vi "Stufen abfragen.vi"(4 "auto Scan Points":bool, 5 "Punkte umkehren":bool, 6 "Sprachliste":string[][](array[string]), 7 "Komponentenauswahl":T9 {"Konzentration" format="%#.6f"}, 8 "error in (no error)":errorcluster caption="Fehler (Eingang, kein Fehler)", 9 "Index Cluster":T7 {"Verdünnungsgas" items=["N2", "O2"]; "Anzahl Stufen" format="%#_5g"}, 10 "Bollche Flags Cluster":T2, 11 "GD Info Cluster":T1) -> (0 "error out":errorcluster caption="Fehler (Ausgang)", 1 "Komponente out":T8, 2 "Status out":string, 3 "GD out":T4)   [LabVIEW 2020, in "Linearisierung v2.lvlib" / "Gasteiler.lvlib"]
uses:
  Gasteiler.lvlib
  KomponentenArray.ctl
  Visualisierungs Elemente/Auswahlfeld.ctl
  Visualisierungs Elemente/Zahlen-Eingabefeld.ctl
  Seiten/System Einstellungen V2/Traegergas.ctl
  Aktionen FGV Gasteiler Daten.ctl
  Aktion FGV Gasteilerliste laden.ctl
  SpanEinstellungen/Aktion FGV GD Errors sammeln.ctl
  SpanEinstellungen/GD Info Cluster.ctl
  LIN ErrorCluster.ctl
  AK-Komm Gasteiler/Aktionen AK Komm.ctl
  AK-Komm Gasteiler/Alter Gasteiler/Aktionen AK Komm_ALT.ctl
  Horiba/Aktion Befehl.ctl
  Gasteiler Fehler.ctl
  Aktion FGV Gasteiler Korrektur.ctl
  AK-Komm Gasteiler/AK Komm Gasteiler.lvlib
  Aktion Lin Daten aufarbeiten.ctl
  Linearisierung v2.lvlib
  AK-Komm Gasteiler/Alter Gasteiler/Alter Gasteiler.lvlib
  Horiba/Horiba GDC.lvlib
  SpanEinstellungen/SpanEinstellungen.lvlib
  HovaCal/HovaCal.lvlib
  Seiten/System Einstellungen V2/System Einstellungen V2.lvlib
  HovaCAL_Interface/HovaCAL_Interface.lvlib
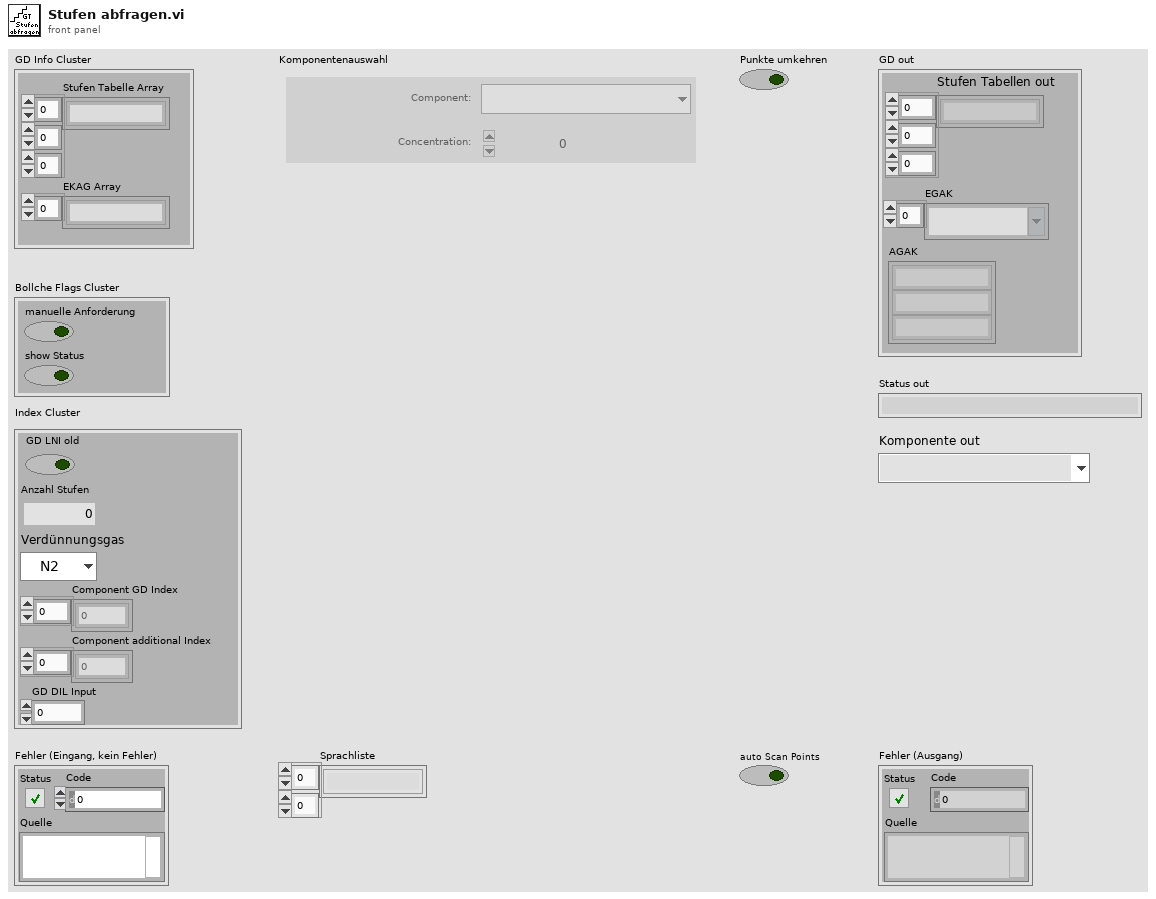
[diagram p1: front panel]
types:
  T1 = cluster{"Stufen Tabelle Array":string[][][], "EKAG Array":string[]}
  T2 = cluster{"manuelle Anforderung":bool, "show Status":bool}
  T3 = typedef "System Einstellungen V2.lvlib/Traegergas.ctl" = string
  T4 = cluster{"Stufen Tabellen out":string[][][], "EGAK":T3[], "AGAK":string[]}
  T5 = typedef "Zahlen-Eingabefeld.ctl" = sgl
  T6 = typedef "Linearisierung v2.lvlib/Gasteiler.lvlib/Prüfgas in.ctl" = u16
  T7 = cluster{"GD LNI old":bool, "Anzahl Stufen":T5, "Verdünnungsgas":T6, "Component GD Index":i32[], "Component additional Index ":i32[], "GD DIL Input":u16}
  T8 = typedef "Auswahlfeld.ctl" = u16
  T9 = typedef "Linearisierung v2.lvlib/KomponentenArray.ctl" = cluster{"Komponente:":T8, "Konzentration":dbl}[]
  T10 = typedef "Linearisierung v2.lvlib/Gasteiler.lvlib/Aktionen FGV Gasteiler Daten.ctl" = enum16{"lesen", "Gasteiler Daten", "Seriellen Param.", "MB-Endwert", "laden", "speichern", "Anforderung", "TCP", "Aufzeichnung Start"}
  T11 = typedef "Linearisierung v2.lvlib/Aktion Lin Daten aufarbeiten.ctl" = enum16{"lesen", "Protkolldaten", "speichern", "laden", "EPA auswerten", "Tabelle schreiben", "Lin auswerten", "Tab init", "Stufentabelle", "EPA aktiviert", "Nachbehandlung laden", "Tabelle löschen", "Istwerte löschen", "Zeile löschen", "Zeile einfügen", "LIN aktiviert", "LIN/EPA aktiv laden", "EGAK Tab", "LIN übernehmen", "Tab init ohne Stufen"}
  T12 = typedef "Linearisierung v2.lvlib/Lin-Polynom Daten.ctl" = cluster{"Messgerät":string, "Kalibrator (Gasteiler)":string, "Bearbeiter/in":string, "Komponente":string, "Zeitstempel":timestamp, "F_max gefordert (%)":sgl, "F_max in %":sgl, "F_max in ppm":sgl, "Vorschlag Ordnung":i32, "Polynom OK":bool, "Polynomkoeff.":dbl[], "Prüfgas Konzentration":dbl, "Pfad EPA":string, "Pfad_LIN":string, "Gasnummer:":u8, "Komponentenauswahl":T9, "Verdünnungsgas":T6, "Zeitdauer Stufe":T5, "Anzahl Stufen":T5, "F_max in % EPA":sgl, "F_max in ppm EPA":sgl, "F_max in % LIN":sgl, "F_max in ppm LIN":sgl, "Punkte umkehren":bool, "EPA Optionsfeld":T13, "Autolin Hovacal":T14, "Spanfactors":sgl[], "Kalibrierauswahl":T15, "Conditions:":T16, "Gasflaschen Nr.:":string, "Bottle Accuracy":dbl, "Konfig Gasflasche":T17, "Gasflasche":T18, "HovaCAL Flow AutoLin":T19, "MFC Output":T20, "Gas Ablaufdatum":timestamp, "Lin Modus":T21, "zusätzliche Zeitdauer Erster Punkt":sgl, "Offsets":sgl[]}
  T13 = typedef "Linearisierung v2.lvlib/EPA Optionsfeld.ctl" = enum32{"Istwert", "Rohwert", "Linearisierter Wert"}
  T14 = typedef "Linearisierung v2.lvlib/Gasteiler.lvlib/HovaCal.lvlib/AutoLin Hovacal.ctl" = enum32{"Keine Auswahl", "Optionsauswahl 1", "Optionsauswahl 2"}
  T15 = typedef "Linearisierung v2.lvlib/Kalibrieroption.ctl" = u16
  T16 = typedef "Linearisierung v2.lvlib/Linearity verification 1065-307.lvlib/Condition.ctl" = u16
  T17 = typedef "System Einstellungen V2.lvlib/Konfig Gasflasche.ctl" = bool
  T18 = typedef "System Einstellungen V2.lvlib/Gasflasche Auswahl.ctl" = u16
  T19 = typedef "Linearisierung v2.lvlib/Gasteiler.lvlib/HovaCAL_Interface.lvlib/Controls.lvlib/Flow Einstellung.ctl" = cluster{"HovaCAL Flow Input Cluster":dbl}
  T20 = typedef "Linearisierung v2.lvlib/Gasteiler.lvlib/HovaCAL_Interface.lvlib/Controls.lvlib/Pump state.ctl" = cluster{"Run":bool}
  T21 = typedef "Linearisierung v2.lvlib/Lin Modus.ctl" = u16
  T22 = typedef "Linearisierung v2.lvlib/Gasteiler.lvlib/Aktion FGV Gasteilerliste laden.ctl" = enum16{"lesen", "laden", "speichern", "Liste erstellen", "Formel ändern", "Gas vereinzeln"}
  T23 = typedef "Linearisierung v2.lvlib/Gasteiler.lvlib/Gasteiler Daten.ctl" = cluster{"Gasteiler":T24, "Gasteiler Stufen":T25, "Gasteiler Type":T26, "Konfig Gasteiler":T27, "Gasteiler Span Eingänge":u16}
  T24 = typedef "String - Eingabefeld.ctl" = string
  T25 = typedef "Linearisierung v2.lvlib/Gasteiler.lvlib/Gasteiler Stufen.ctl" = u16
  T26 = typedef "Linearisierung v2.lvlib/GasteilerType.ctl" = u16
  T27 = typedef "System Einstellungen V2.lvlib/Gasteiler Auswahl.ctl" = u16
  T28 = typedef "Linearisierung v2.lvlib/SpanEinstellungen.lvlib/GD Info Cluster.ctl" = cluster{"Wobei":string, "Status":string, "Errors":T29, "Empfangsdaten":string[], "Zeitstempel":string}
  T29 = typedef "Linearisierung v2.lvlib/LIN ErrorCluster.ctl" = cluster{"Störung Kommunikation":bool, "Pressure carrier gas":bool, "Pressure diluted gas":bool, "Outlet Pressure":bool, "SNOX before SAIR":bool, "Störung Gasteiler":bool}
  T30 = typedef "Linearisierung v2.lvlib/SpanEinstellungen.lvlib/Aktion FGV GD Errors sammeln.ctl" = enum16{"lesen", "init", "GD Infos sammeln", "Kalibrierinfos sammeln", "Test Data", "GD Infos selektiv sammeln"}
  T31 = typedef "Linearisierung v2.lvlib/Gasteiler.lvlib/AK Komm Gasteiler.lvlib/Aktionen AK Komm.ctl" = enum16{"lesen", "initialisieren", "beenden", "Status", "SMAN", "SREM", "STBY", "ASTF", "ASTZ", "SLST", "AGAT", "EGAK", "AGAK", "AKAK", "ADRU", "SKOP", "SVSA", "SVSZ", "SONO", "SAIR", "SNOX", "ANOX", "SSPL", "SRUC", "SLIN", "ALST", "ETYP", "SVIO", "LCYL", "CCYL", "DCYL", "SCYL", "GCYL", "DRGV", "DRDC"}
  T32 = typedef "Linearisierung v2.lvlib/Gasteiler.lvlib/AK Komm Gasteiler.lvlib/Alter Gasteiler.lvlib/Aktionen AK Komm_ALT.ctl" = enum16{"lesen", "initialisieren", "beenden", "SRES", "STBY", "SREM", "SMAN", "SLIN", "SLCH", "SLST", "SSPL", "AGAT", "ALST", "ASTZ", "ASTF", "AGAK", "EGAK"}
  T33 = typedef "Linearisierung v2.lvlib/Gasteiler.lvlib/Gasteiler Fehler.ctl" = cluster{"Pressure carrier gas":bool, "Pressure diluted gas":bool, "Outlet Pressure":bool, "SNOX before SAIR":bool}
  T34 = typedef "Linearisierung v2.lvlib/Gasteiler.lvlib/Horiba GDC.lvlib/Aktion Befehl.ctl" = enum16{"lesen", "initialisieren", "Beenden", "Standby", "GD/CC", "Info", "Flow", "Alarm", "GD parameter", "GD point", "Durchfluss", "Spuelen1", "Spuelen1 On", "Spuelen1Off", "Spuelen2", "Ventil-Abfrage", "Reset"}
  T35 = typedef "Linearisierung v2.lvlib/Gasteiler.lvlib/Aktion FGV Gasteiler Korrektur.ctl" = enum16{"lesen", "schreiben", "laden", "speichern", "B-nr und Gültig", "Gasteilernr.", "Vereinzeln", "aktiv"}
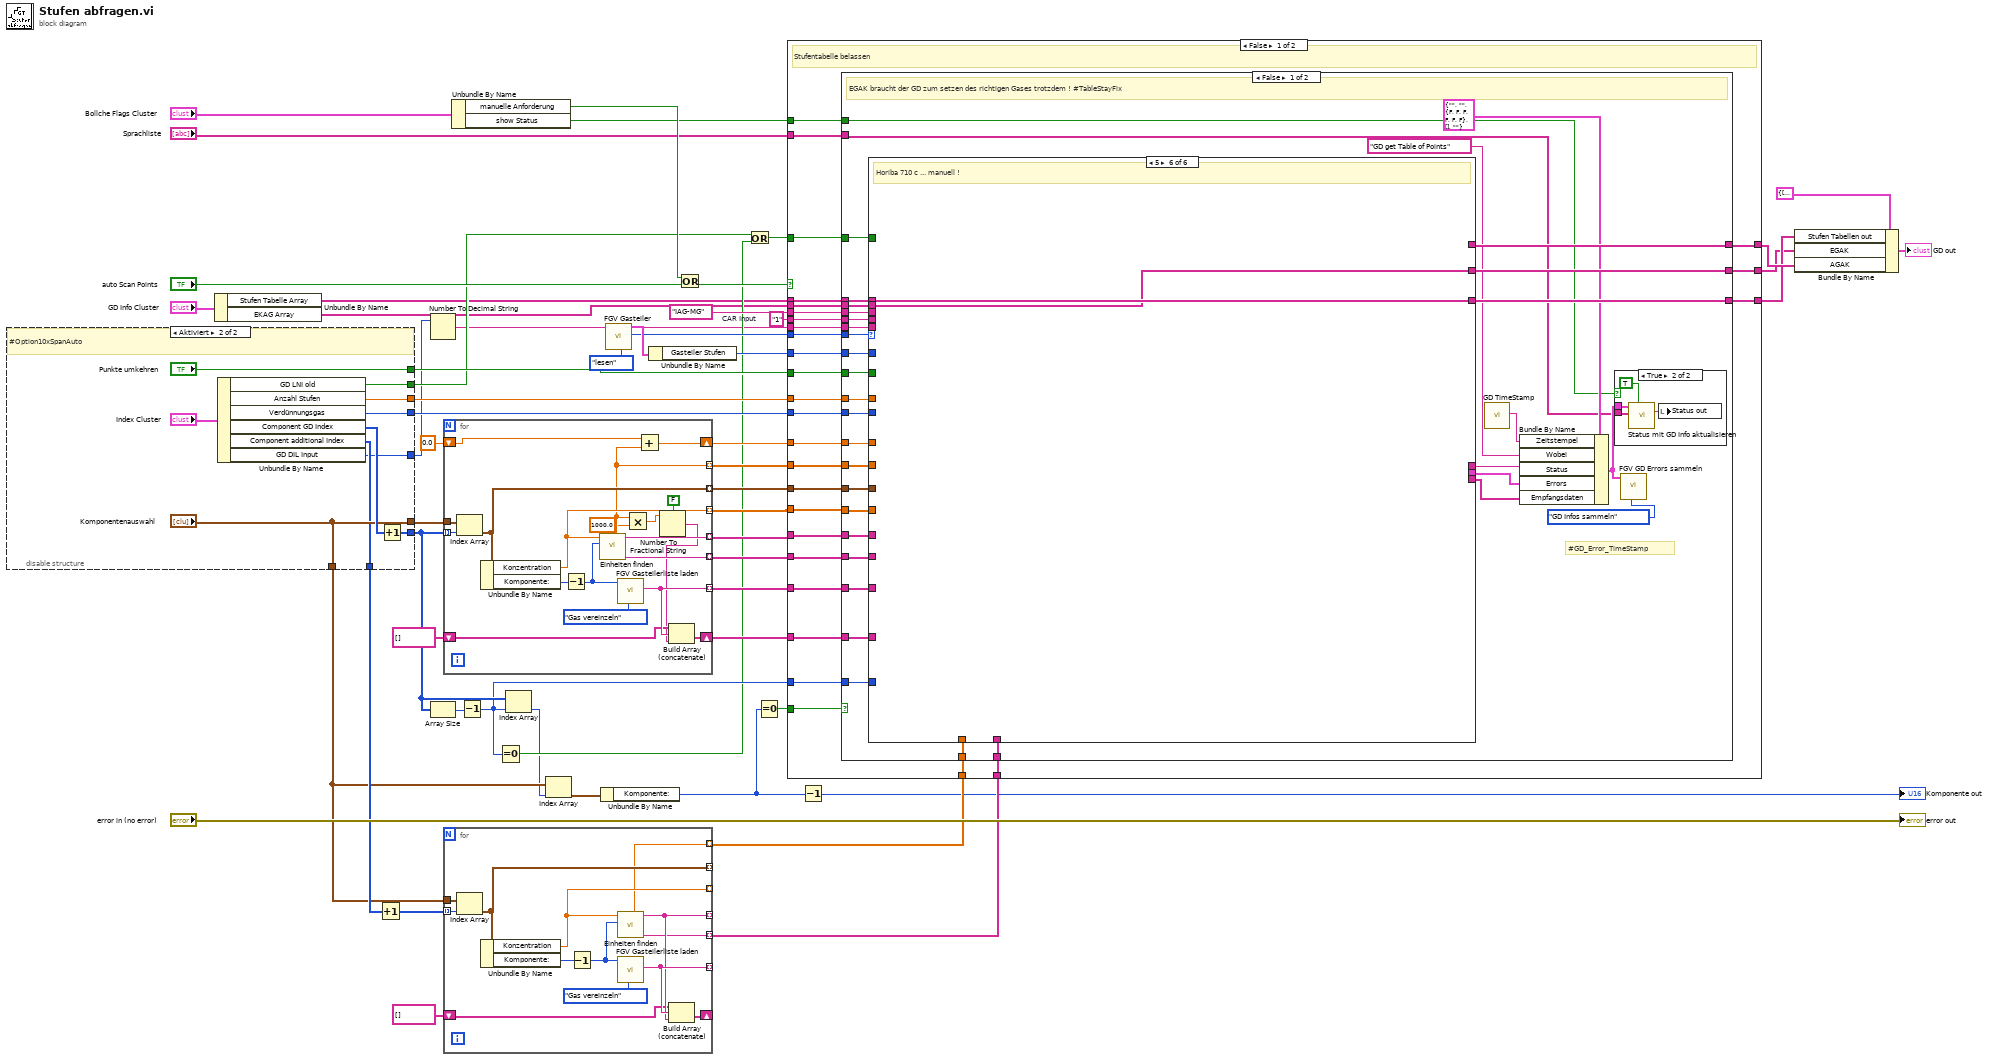
[diagram p0: block diagram]
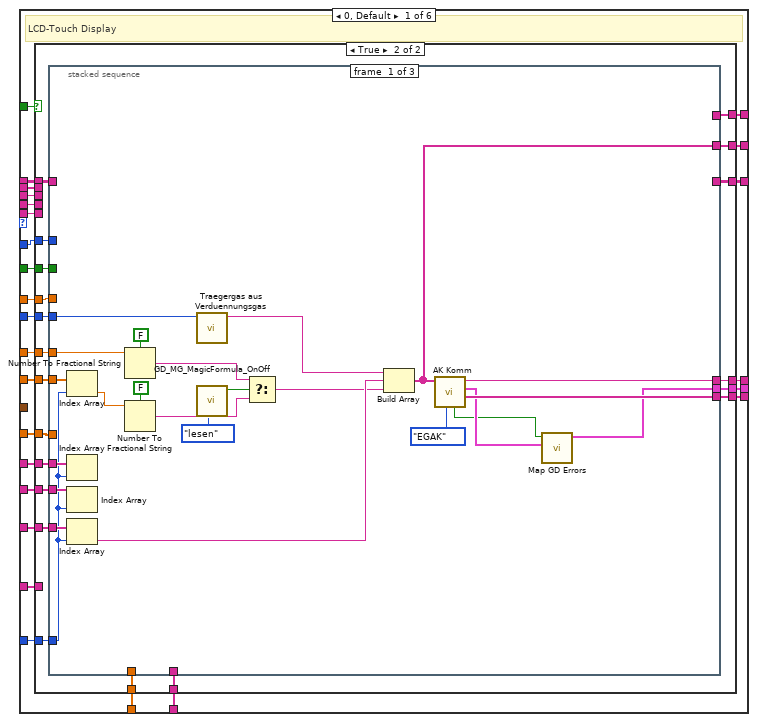
[diagram p2: hidden frame]
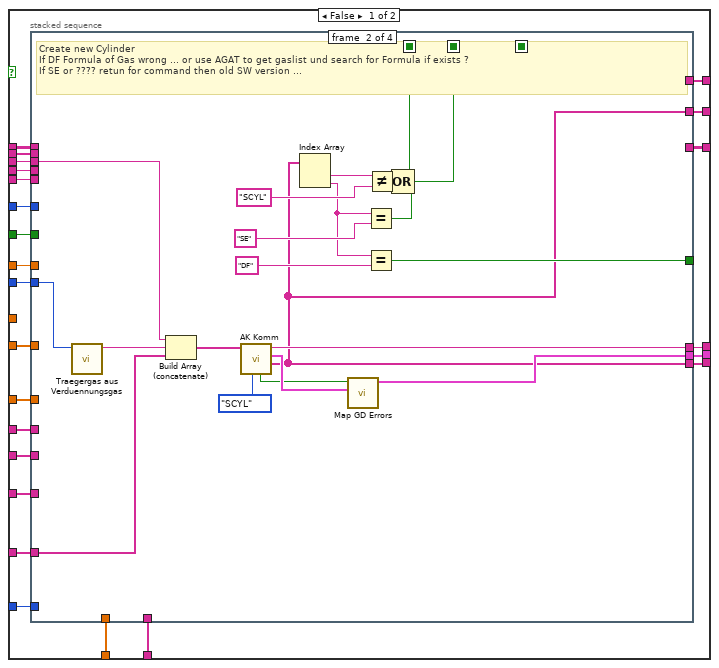
[diagram p3: hidden frame]
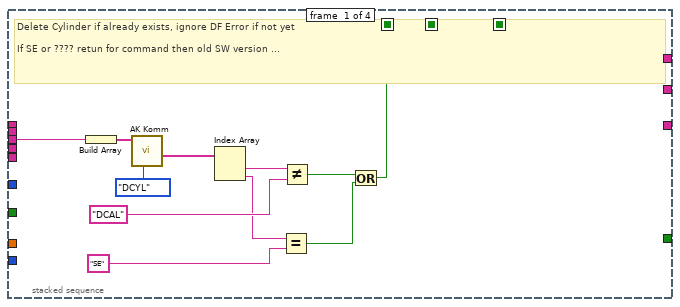
[diagram p4: hidden frame]
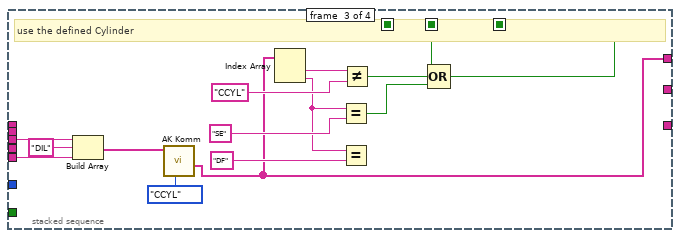
[diagram p5: hidden frame]
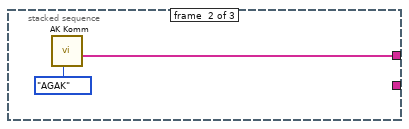
[diagram p7: hidden frame]
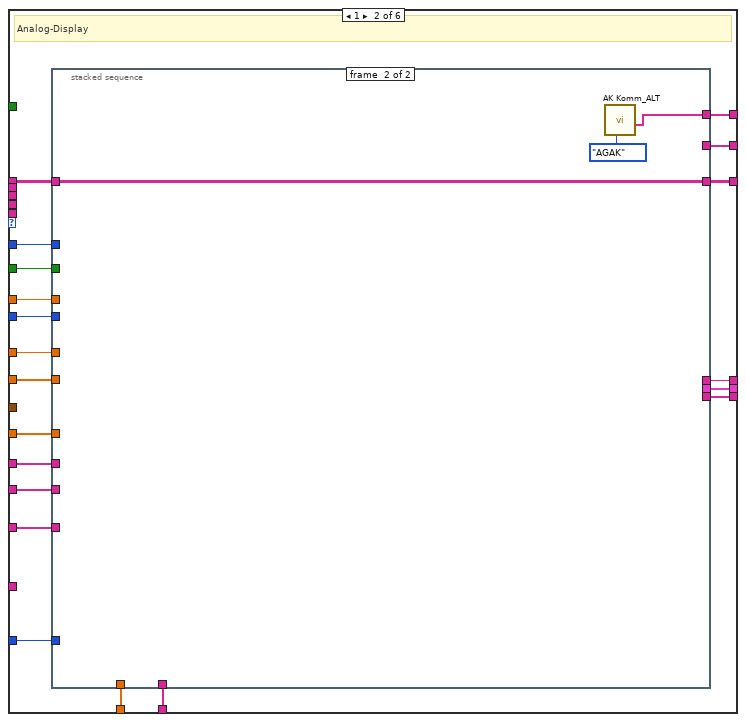
[diagram p9: hidden frame]
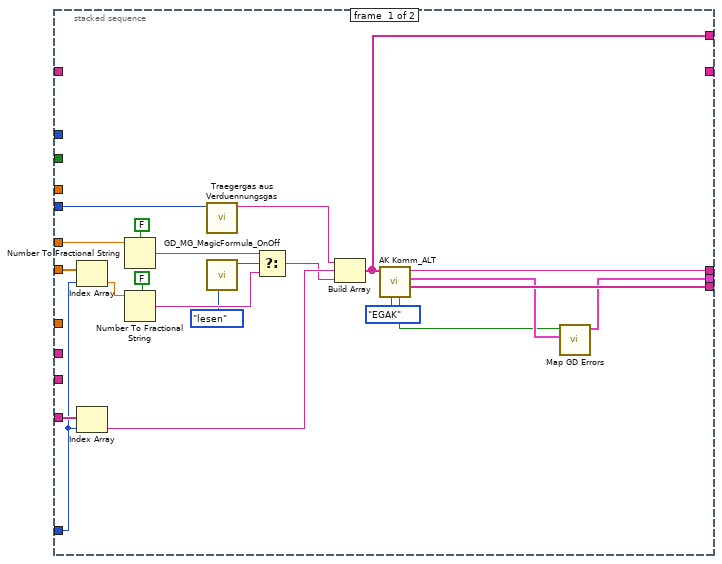
[diagram p10: hidden frame]
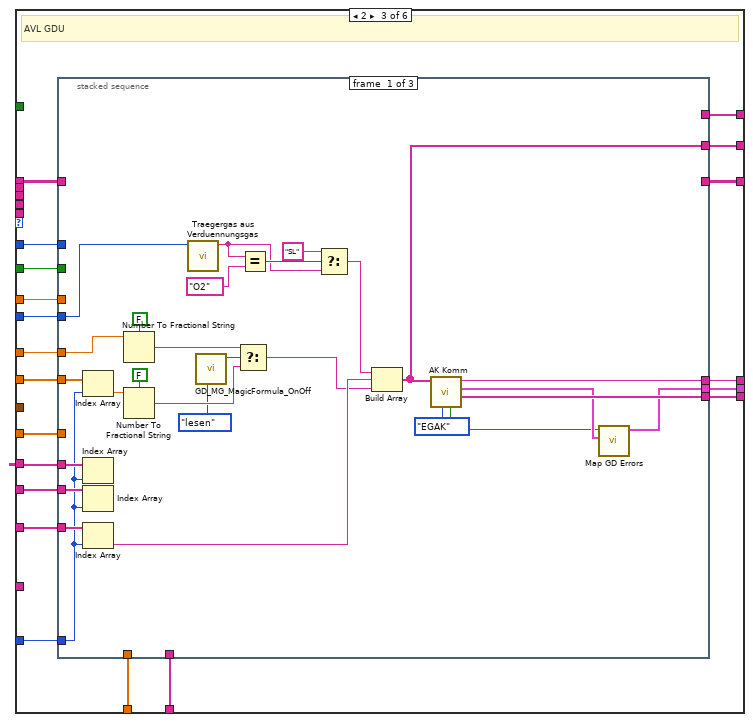
[diagram p11: hidden frame]
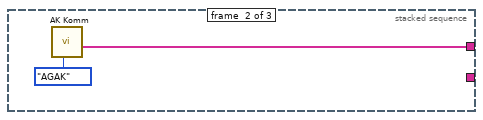
[diagram p12: hidden frame]
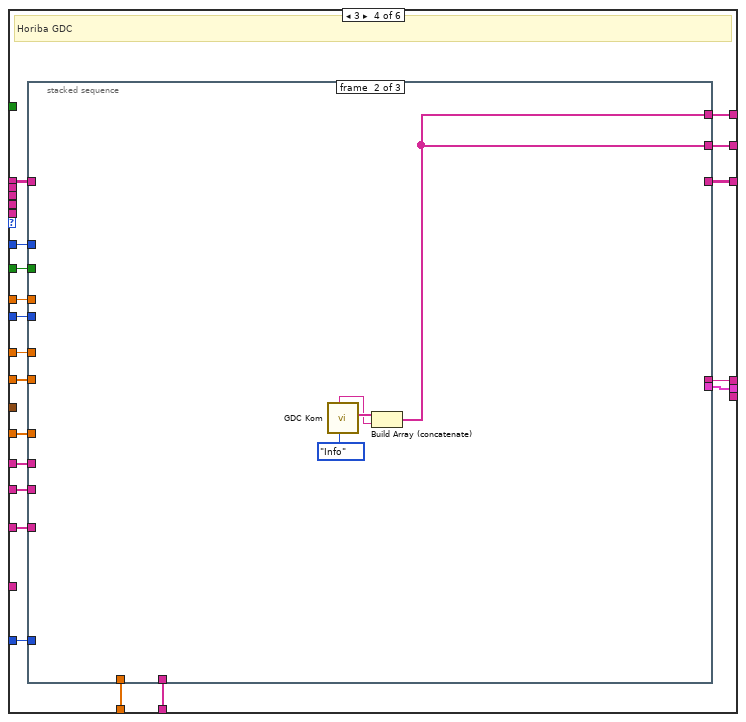
[diagram p14: hidden frame]
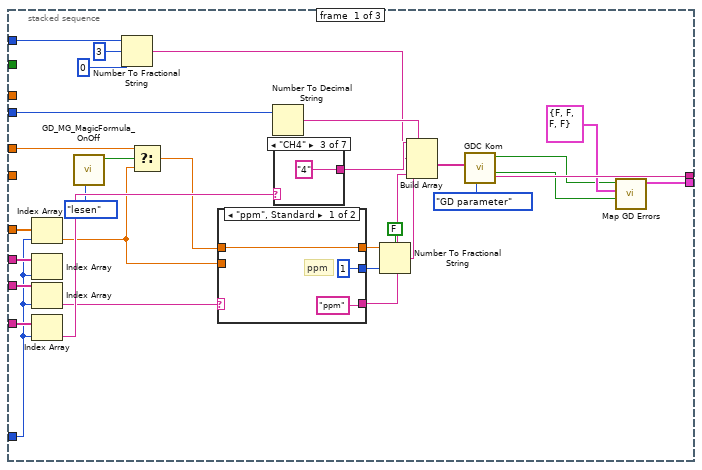
[diagram p15: hidden frame]
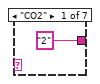
[diagram p16: hidden frame]
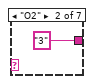
[diagram p17: hidden frame]
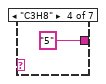
[diagram p18: hidden frame]
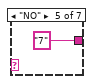
[diagram p19: hidden frame]
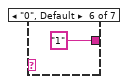
[diagram p20: hidden frame]
diagram:
  w6 = "1"  # CAR Input
  n1 = disable-structure shown="Aktiviert" {
    disable-tunnel: [w62 "Komponentenauswahl"] -> w36
    disable-tunnel: [w61 w70] -> w53
    disable-tunnel: [w59 w71] -> w52
    disable-tunnel: [w56 "Punkte umkehren"] -> w51
    disable-tunnel: [w55 w68] -> w26
    disable-tunnel: [_ w67] -> w31
    disable-tunnel: [_ "Komponentenauswahl"] -> w11
    disable-tunnel: [_ w65] -> w20
    disable-tunnel: [_ w64] -> w5
    frame Disabled {
      n2 = call "Lin Daten aufarbeiten.vi"("Aktionen"=Aktion_Lin_Daten_aufarbeiten."lesen") -> ("Lin-Polynom"=w60:T12)  [unwired: 16 in, 10 out]
      n3 = call "Lin Daten aufarbeiten.vi"("Aktionen"=Aktion_Lin_Daten_aufarbeiten."lesen") -> ("Lin-Polynom"=w57:T12)  [unwired: 16 in, 10 out]
      n4 = Unbundle By Name(w60) -> ("Komponentenauswahl"=w62:T9, "Gasnummer:"=w55:u8)
      n5 = Unbundle By Name(w60) -> ("Verdünnungsgas"=w61:T6, "Anzahl Stufen"=w59:T5)
      n6 = Unbundle By Name(w57) -> ("Punkte umkehren"=w56:bool)
    }
    frame Enabled {
      # "#Option10xSpanAuto"
      n7 = Unbundle By Name("Index Cluster") -> ("GD LNI old"=w67:bool, "Anzahl Stufen"=w71:T5, "Verdünnungsgas"=w70:T6, "Component GD Index"=w69:i32[], "Component additional Index"=w65:i32[], "GD DIL Input"=w64:u16)
      n8 = Increment(x=w69) -> (x+1=w68:i32[])
    }
  }
  n9 = Unbundle By Name("GD Info Cluster") -> ("Stufen Tabelle Array"=w2:string[][][], "EKAG Array"=w1:string[])
  n10 = Increment(x=w20) -> (x+1=w19:i32[])
  n11 = Number To Decimal String(number=w5) -> (decimal integer string=w4:string)  [unwired: 1 in]
  n12 = Array Size(array=w26) -> (size(s)=w25:i32)
  n13 = for {
    tunnel: w36 -> [w92]
    tunnel: w26 -> [w91] mode=indexing
    tunnel: [w86] -> w35 mode=indexing
    tunnel: [w87] -> w27 mode=indexing
    shift-right: [w85] -> w29
    shift-left: string[] [] -> [w84]
    tunnel: [w83] -> w34 mode=indexing
    tunnel: [w82] -> w33 mode=indexing
    tunnel: [w81] -> w32 mode=indexing
    shift-right: [w80] -> w21
    shift-left: 0.0 -> [w79]
    tunnel: [w78] -> w22 mode=indexing
    n14 = Index Array(array=w92, index=w91) -> (element=w81:cluster{"Komponente:":T8, "Konzentration":dbl})
    n15 = Unbundle By Name(w81) -> ("Konzentration"=w82:dbl, "Komponente:"=w89:T8)
    n16 = Decrement(x=w89) -> (x-1=w88:T8)
    n17 = call "Einheiten finden.vi"("Komponente"=w88, "Wert"=w82) -> ("Einheit in String"=w83:string, "String"=w86:string, "Wert ppm"=w78:dbl)  [unwired: 5 in, 2 out]
    n18 = call "FGV Gasteilerliste laden.vi"("Aktion"=Aktion_FGV_Gasteilerliste_laden."Gas vereinzeln", "Gasindex"=w88) -> ("Formel"=w87:string)  [unwired: 7 in, 2 out]
    n19 = Multiply(x=w78, y=1000.0) -> (x*y=w75:dbl)
    n20 = Add(x=w79, y=w78) -> (x+y=w80:dbl)
    n21 = Number To Fractional String(use system decimal point (T)=FALSE ("Systemdezimalzeichen verwenden (T)"), number=w75) -> (F-format string=w74:string)  [unwired: 2 in]
    n22 = Build Array (concatenate)(w84, w87, w74) -> (w85:string[])
  }
  n23 = for {
    tunnel: w11 -> [w105]
    tunnel: w19 -> [w104] mode=indexing
    tunnel: [w99] -> _ mode=indexing
    tunnel: [w100] -> _ mode=indexing
    shift-right: [w98] -> _
    shift-left: string[] [] -> [w97]
    tunnel: [w96] -> w16 mode=indexing
    tunnel: [w95] -> _ mode=indexing
    tunnel: [w94] -> _ mode=indexing
    tunnel: [w93] -> w15 mode=indexing
    n24 = Index Array(array=w105, index=w104) -> (element=w94:cluster{"Komponente:":T8, "Konzentration":dbl})
    n25 = Unbundle By Name(w94) -> ("Konzentration"=w95:dbl, "Komponente:"=w102:T8)
    n26 = Decrement(x=w102) -> (x-1=w101:T8)
    n27 = call "Einheiten finden.vi"("Komponente"=w101, "Wert"=w95) -> ("Einheit in String"=w96:string, "String"=w99:string, "Wert ppm"=w93:dbl)  [unwired: 5 in, 2 out]
    n28 = call "FGV Gasteilerliste laden.vi"("Aktion"=Aktion_FGV_Gasteilerliste_laden."Gas vereinzeln", "Gasindex"=w101) -> ("Formel"=w100:string)  [unwired: 7 in, 2 out]
    n29 = Build Array (concatenate)(w97, w100, w99) -> (w98:string[])
  }
  n30 = Unbundle By Name("Bollche Flags Cluster") -> ("manuelle Anforderung"=w39:bool, "show Status"=w38:bool)
  n31 = Decrement(x=w25) -> (x-1=w13:i32)
  n32 = Equal To 0?(x=w13) -> (x = 0?=w12:bool)
  n33 = Index Array(array=w26, index=w13) -> (element=w10:i32)
  n34 = Index Array(array=w11, index=w10) -> (element=w9:cluster{"Komponente:":T8, "Konzentration":dbl})
  n35 = Unbundle By Name(w9) -> ("Komponente:"=w8:T8)
  n36 = call "FGV Gasteiler.vi"("Aktionen"=Aktionen_FGV_Gasteiler_Daten."lesen") -> ("Gasteiler Daten"=w49:T23, "Gasteiler Type"=w47:T26)  [unwired: 11 in, 6 out]
  n37 = Unbundle By Name(w49) -> ("Gasteiler Stufen"=w46:T25)
  n38 = Or(x=w39, y="auto Scan Points") -> (x .or. y?=w41:bool)
  n39 = Or(x=w31, y=w12) -> (x .or. y?=w14:bool)
  n40 = Equal To 0?(x=w8) -> (x = 0?=w45:bool)
  n41 = case shown="False" w41 {
    tunnel: w53 -> [w118 w522]
    tunnel: w52 -> [w117 w521]
    tunnel: w51 -> [w107 w520]
    tunnel: w2 -> [w112 w519]
    tunnel: [w131 w518] -> w43
    tunnel: w35 -> [w123 w517]
    tunnel: w33 -> [w122 w516]
    tunnel: w47 -> [w108 w515]
    tunnel: w46 -> [w116 w514]
    tunnel: [w132 w513] -> w42
    tunnel: [w133 w512] -> w44
    tunnel: w45 -> [w128 w511]
    tunnel: w38 -> [w114 w510]
    tunnel: "Sprachliste" -> [w113 w509]
    tunnel: w27 -> [w125 w508]
    tunnel: w34 -> [w124 w507]
    tunnel: w32 -> [w121 w506]
    tunnel: w14 -> [w115 w505]
    tunnel: "IAG-MG" -> [w111 w504]
    tunnel: w29 -> [w126 w503]
    tunnel: w21 -> [w119 w502]
    tunnel: w13 -> [w127 w501]
    tunnel: w22 -> [w120 w500]
    tunnel: w15 -> [w129 w499]
    tunnel: w16 -> [w130 w498]
    tunnel: w4 -> [w109 w497]
    tunnel: w6 -> [w110 w496]
    tunnel: w1 -> [w106 w495]
    frame False {
      # "Stufentabelle belassen"
      n42 = case shown="False" w128 {
        tunnel: w108 -> [w168 _]
        tunnel: w122 -> [w167 _]
        tunnel: w116 -> [w166 _]
        tunnel: w118 -> [w165 _]
        tunnel: w117 -> [w164 _]
        tunnel: w107 -> [w163 _]
        tunnel: w112 -> [w159 w494]
        tunnel: [w162 w494] -> w131
        tunnel: [w161 w493] -> w132
        tunnel: [w160 _] -> w133
        tunnel: w114 -> [w151 _]
        tunnel: w113 -> [w150 _]
        tunnel: w125 -> [w149 _]
        tunnel: w121 -> [w148 _]
        tunnel: w115 -> [w147 _]
        tunnel: w111 -> [w146 _]
        tunnel: w126 -> [w145 _]
        tunnel: w119 -> [w144 _]
        tunnel: w127 -> [w143 _]
        tunnel: w120 -> [w142 _]
        tunnel: w129 -> [w141 _]
        tunnel: w130 -> [w140 _]
        tunnel: w109 -> [w139 _]
        tunnel: w110 -> [w138 _]
        tunnel: w124 -> [w135 _]
        tunnel: w123 -> [w136 _]
        tunnel: w106 -> [w134 w493]
        frame False {
          # "#GD_Error_TimeStamp"
          # "EGAK braucht der GD zum setzen des richtigen Gases trotzdem ! #TableStayFix"
          n43 = case shown="5" w168 {
            tunnel: w136 -> [w194 w333 w378 w427 _ _]
            tunnel: w167 -> [w193 w332 w377 w426 _ _]
            tunnel: w166 -> [w192 w331 w366 w428 _ _]
            tunnel: w165 -> [w191 w329 w360 w424 _ _]
            tunnel: w164 -> [w190 w330 w376 w425 _ _]
            tunnel: w163 -> [w189 w328 w375 w423 _ _]
            tunnel: [w188 w316 w361 w411 w486 w488] -> w162
            tunnel: [w187 w327 w373 w422 w485 w487] -> w161
            tunnel: [w186 w315 w374 w421 _ _] -> w160
            tunnel: w159 -> [w170 w314 w359 w410 w486 w488]
            tunnel: [w185 w326 w372 w420 _ _] -> w155
            tunnel: [w184 w324 w370 w419 _ _] -> w154
            tunnel: [w178 w325 w371 _ _ _] -> w153
            tunnel: w149 -> [w183 w322 w369 w418 _ _]
            tunnel: w135 -> [w182 w323 w368 w417 _ _]
            tunnel: w148 -> [_ _ _ _ _ _]
            tunnel: w147 -> [w181 _ _ _ _ _]
            tunnel: w146 -> [w180 _ _ _ _ _]
            tunnel: w145 -> [w179 _ _ _ _ _]
            tunnel: w144 -> [w177 w317 w365 w415 _ _]
            tunnel: w143 -> [w176 w321 w367 w416 _ _]
            tunnel: w142 -> [w175 w319 w363 w412 _ _]
            tunnel: w141 -> [w174 w320 w364 w414 _ _]
            tunnel: w140 -> [w173 w318 w362 w413 _ _]
            tunnel: w139 -> [w172 _ _ _ _ _]
            tunnel: w138 -> [w171 _ _ _ _ _]
            tunnel: w134 -> [w169 _ _ _ w485 w487]
            frame 0, Default {
              # "LCD-Touch Display"
              n44 = case shown="True" w181 {
                tunnel: w194 -> [w218 w286]
                tunnel: w193 -> [w216 w285]
                tunnel: w192 -> [w208 w284]
                tunnel: w191 -> [w213 w283]
                tunnel: w190 -> [w215 w282]
                tunnel: w189 -> [w207 w281]
                tunnel: [w203 w280] -> w188
                tunnel: [w206 w279] -> w187
                tunnel: [w205 w278] -> w186
                tunnel: [w211 w277] -> w185
                tunnel: [w210 w275] -> w184
                tunnel: w183 -> [w204 w274]
                tunnel: w182 -> [w217 w273]
                tunnel: w180 -> [w214 _]
                tunnel: w179 -> [w212 _]
                tunnel: [w209 w276] -> w178
                tunnel: w177 -> [_ w269]
                tunnel: w176 -> [w199 w272]
                tunnel: w175 -> [w200 w268]
                tunnel: w174 -> [w202 w271]
                tunnel: w173 -> [w201 w270]
                tunnel: w172 -> [w198 _]
                tunnel: w171 -> [w197 _]
                tunnel: w170 -> [w196 w267]
                tunnel: w169 -> [w195 _]
                frame False {
                  n45 = stacked-sequence {
                    seq-local: [w219 _ _ _] -> [_ w233 _ _]
                    seq-local: [_ w232 _ _] -> [_ _ w254 _]
                    seq-local: [_ _ w253 _] -> [_ _ _ _]
                    tunnel: w217 -> [_ _ _ _]
                    tunnel: w216 -> [_ _ _ _]
                    tunnel: [_ w247 _ _] -> w211
                    tunnel: [_ w230 _ _] -> w209
                    tunnel: [_ w245 _ _] -> w210
                    tunnel: w214 -> [w228 w243 w263 _]
                    tunnel: w212 -> [_ w242 _ _]
                    tunnel: [_ w234 _ _] -> _
                    tunnel: w218 -> [_ _ _ _]
                    tunnel: w215 -> [_ _ _ _]
                    tunnel: w213 -> [_ w231 _ _]
                    tunnel: w208 -> [_ _ _ _]
                    tunnel: w207 -> [_ _ _ _]
                    tunnel: [_ w230 _ _] -> w206
                    tunnel: [_ _ w252 _] -> w205
                    tunnel: w204 -> [_ _ _ _]
                    tunnel: [_ _ _ w266] -> w203
                    tunnel: w202 -> [_ _ _ _]
                    tunnel: w201 -> [_ _ _ _]
                    tunnel: w200 -> [_ _ _ _]
                    tunnel: w199 -> [_ _ _ _]
                    tunnel: w198 -> [_ _ w251 _]
                    tunnel: w197 -> [_ _ _ _]
                    tunnel: w196 -> [_ _ _ w266]
                    tunnel: w195 -> [_ _ _ _]
                    frame #0 {
                      # "Delete Cylinder if already exists, ignore DF Error if not yet\n\nIf SE or ???? retun for command then old SW version ..."
                      n46 = Build Array(w228) -> (w227:string[])
                      n47 = call "AK Komm.vi"("Aktionen"=Aktionen_AK_Komm."DCYL", "Daten"=w227) -> ("Empfangsdaten"=w226:string[])  [unwired: 3 in, 6 out]
                      n48 = Index Array(array=w226) -> (element #1=w225:string, element #2=w222:string)  [unwired: 2 in]
                      n49 = Equal?(x=w222, y="SE") -> (x = y?=w220:bool)
                      n50 = Not Equal?(x=w225, y="DCAL") -> (x != y?=w223:bool)
                      n51 = Or(x=w223, y=w220) -> (x .or. y?=w219:bool)
                    }
                    frame #1 {
                      # "Create new Cylinder \nIf DF Formula of Gas wrong ... or use AGAT to get gaslist und search for Formula if exists ?\nIf SE or ???? retun for command then old SW version ..."
                      n52 = call "Traegergas aus Verduennungsgas.vi"("Verdünnungsgas"=w231) -> ("Trägergas"=w249:T3)  [unwired: 10 in]
                      n53 = Build Array (concatenate)(w243, w249, w242) -> (w248:T3[])
                      n54 = call "AK Komm.vi"("Aktionen"=Aktionen_AK_Komm."SCYL", "Daten"=w248) -> ("Empfangsdaten"=w230:string[], "Error"=w246:T33, "Status"=w247:string, "Störung Kommunikation"=w244:bool)  [unwired: 3 in, 3 out]
                      n55 = Index Array(array=w230) -> (element #1=w241:string, element #2=w238:string)  [unwired: 2 in]
                      n56 = call "Map GD Errors.vi"("Error"=w246, "Störung Kommunikation"=w244) -> ("LIN Errors-Cluster (Ausgang)"=w245:T29)  [unwired: 8 in, 1 out]
                      n57 = Equal?(x=w238, y="SE") -> (x = y?=w235:bool)
                      n58 = Equal?(x=w238, y="DF") -> (x = y?=w234:bool)
                      n59 = Not Equal?(x=w241, y="SCYL") -> (x != y?=w236:bool)
                      n60 = Compound Arithmetic op=OR ("Mehrfacharithmetik")(w233, w236, w235) -> (w232:bool)
                    }
                    frame #2 {
                      # "use the defined Cylinder"
                      n61 = Build Array(w263, "DIL", w251) -> (w264:string[])
                      n62 = call "AK Komm.vi"("Aktionen"=Aktionen_AK_Komm."CCYL", "Daten"=w264) -> ("Empfangsdaten"=w252:string[])  [unwired: 3 in, 6 out]
                      n63 = Index Array(array=w252) -> (element #1=w261:string, element #2=w258:string)  [unwired: 2 in]
                      n64 = Equal?(x=w258, y="SE") -> (x = y?=w255:bool)
                      n65 = Equal?(x=w258, y="DF") -> ()  [unwired: 1 out]
                      n66 = Not Equal?(x=w261, y="CCYL") -> (x != y?=w256:bool)
                      n67 = Compound Arithmetic op=OR ("Mehrfacharithmetik")(w254, w256, w255) -> (w253:bool)
                    }
                    frame #3 {
                      # "Get a point for all components in cylinder ...\n\nDRGV 0 N2 TestUnit 9 CO2 1.729 N2 9.983E+08 NO2 1.729 O2 1.642E+06"
                    }
                  }
                }
                frame True {
                  n68 = stacked-sequence {
                    tunnel: w286 -> [w299 _ _]
                    tunnel: w285 -> [_ _ _]
                    tunnel: w284 -> [_ _ _]
                    tunnel: w283 -> [w309 _ _]
                    tunnel: w282 -> [_ _ _]
                    tunnel: w281 -> [_ _ _]
                    tunnel: [_ _ w313] -> w280
                    tunnel: [w307 _ _] -> w279
                    tunnel: [_ w311 _] -> w278
                    tunnel: [w306 _ _] -> w277
                    tunnel: [w305 _ _] -> w276
                    tunnel: [w303 _ _] -> w275
                    tunnel: w274 -> [w301 _ _]
                    tunnel: w273 -> [w298 _ _]
                    tunnel: w272 -> [w297 _ _]
                    tunnel: w271 -> [_ _ _]
                    tunnel: w270 -> [_ _ _]
                    tunnel: w269 -> [w295 _ _]
                    tunnel: w268 -> [w291 _ _]
                    tunnel: w267 -> [_ _ w313]
                    frame #0 {
                      n69 = Index Array(array=w291, index=w297) -> (element=w289:dbl)
                      n70 = Index Array(array=w299, index=w297) -> ()  [unwired: 1 out]
                      n71 = Index Array(array=w298, index=w297) -> ()  [unwired: 1 out]
                      n72 = Index Array(array=w301, index=w297) -> (element=w300:string)
                      n73 = Number To Fractional String(use system decimal point (T)=FALSE ("Systemdezimalzeichen verwenden (T)"), number=w295) -> (F-format string=w293:string)  [unwired: 2 in]
                      n74 = Number To Fractional String(use system decimal point (T)=FALSE ("Systemdezimalzeichen verwenden (T)"), number=w289) -> (F-format string=w288:string)  [unwired: 2 in]
                      n75 = call "Traegergas aus Verduennungsgas.vi"("Verdünnungsgas"=w309) -> ("Trägergas"=w308:T3)  [unwired: 10 in]
                      n76 = call "GD_MG_MagicFormula_OnOff.vi"("Aktion"=enum16{"lesen", "schreiben", "init"}."lesen") -> ("MG_use_magic_formula"=w294:bool)  [unwired: 8 in, 1 out]
                      n77 = Select(t=w293, s=w294, f=w288) -> (s? t:f=w292:string)
                      n78 = Build Array(w308, w300, w292) -> (w307:T3[])
                      n79 = call "AK Komm.vi"("Aktionen"=Aktionen_AK_Komm."EGAK", "Daten"=w307) -> ("Empfangsdaten"=w305:string[], "Error"=w304:T33, "Status"=w306:string, "Störung Kommunikation"=w302:bool)  [unwired: 3 in, 3 out]
                      n80 = call "Map GD Errors.vi"("Error"=w304, "Störung Kommunikation"=w302) -> ("LIN Errors-Cluster (Ausgang)"=w303:T29)  [unwired: 8 in, 1 out]
                    }
                    frame #1 {
                      n81 = call "AK Komm.vi"("Aktionen"=Aktionen_AK_Komm."AGAK") -> ("Empfangsdaten"=w311:string[])  [unwired: 4 in, 6 out]
                    }
                    frame #2 {
                    }
                  }
                }
              }
            }
            frame 1 {
              # "Analog-Display"
              n82 = stacked-sequence {
                tunnel: w333 -> [_ _]
                tunnel: w332 -> [_ _]
                tunnel: w331 -> [_ _]
                tunnel: w330 -> [_ _]
                tunnel: w329 -> [w354 _]
                tunnel: w328 -> [_ _]
                tunnel: [_ w356] -> w316
                tunnel: [w352 _] -> w327
                tunnel: [w351 _] -> w326
                tunnel: [w348 _] -> w324
                tunnel: [w350 _] -> w325
                tunnel: w323 -> [_ _]
                tunnel: w322 -> [w346 _]
                tunnel: w321 -> [w344 _]
                tunnel: w320 -> [_ _]
                tunnel: w319 -> [w338 _]
                tunnel: w318 -> [_ _]
                tunnel: w317 -> [w342 _]
                tunnel: [_ w357] -> w315
                tunnel: w314 -> [_ w356]
                frame #0 {
                  n83 = Index Array(array=w338, index=w344) -> (element=w337:dbl)
                  n84 = Index Array(array=w346, index=w344) -> (element=w345:string)
                  n85 = Number To Fractional String(use system decimal point (T)=FALSE ("Systemdezimalzeichen verwenden (T)"), number=w342) -> (F-format string=w340:string)  [unwired: 2 in]
                  n86 = Number To Fractional String(use system decimal point (T)=FALSE ("Systemdezimalzeichen verwenden (T)"), number=w337) -> (F-format string=w335:string)  [unwired: 2 in]
                  n87 = call "Traegergas aus Verduennungsgas.vi"("Verdünnungsgas"=w354) -> ("Trägergas"=w353:T3)  [unwired: 10 in]
                  n88 = call "GD_MG_MagicFormula_OnOff.vi"("Aktion"=enum16{"lesen", "schreiben", "init"}."lesen") -> ("MG_use_magic_formula"=w341:bool)  [unwired: 8 in, 1 out]
                  n89 = Select(t=w340, s=w341, f=w335) -> (s? t:f=w339:string)
                  n90 = Build Array(w353, w345, w339) -> (w352:T3[])
                  n91 = call "AK Komm_ALT.vi"("Aktionen_ALT"=Aktionen_AK_Komm_ALT."EGAK", "Daten"=w352) -> ("Empfangsdaten"=w350:string[], "Error"=w349:T33, "Status"=w351:string, "Störung Kommunikation"=w347:bool)  [unwired: 5 in, 1 out]
                  n92 = call "Map GD Errors.vi"("Error"=w349, "Störung Kommunikation"=w347) -> ("LIN Errors-Cluster (Ausgang)"=w348:T29)  [unwired: 8 in, 1 out]
                }
                frame #1 {
                  n93 = call "AK Komm_ALT.vi"("Aktionen_ALT"=Aktionen_AK_Komm_ALT."AGAK") -> ("Empfangsdaten"=w357:string[])  [unwired: 6 in, 4 out]
                }
              }
            }
            frame 2 {
              # "AVL GDU"
              n94 = stacked-sequence {
                tunnel: w366 -> [_ _ _]
                tunnel: w378 -> [w392 _ _]
                tunnel: w377 -> [_ _ _]
                tunnel: w376 -> [_ _ _]
                tunnel: w375 -> [_ _ _]
                tunnel: [_ w407 _] -> w374
                tunnel: [_ _ w409] -> w361
                tunnel: [w400 _ _] -> w373
                tunnel: [w399 _ _] -> w372
                tunnel: [w398 _ _] -> w371
                tunnel: [w395 _ _] -> w370
                tunnel: w369 -> [w394 _ _]
                tunnel: w368 -> [w391 _ _]
                tunnel: w367 -> [w389 _ _]
                tunnel: w365 -> [w382 _ _]
                tunnel: w364 -> [_ _ _]
                tunnel: w363 -> [w390 _ _]
                tunnel: w362 -> [_ _ _]
                tunnel: w360 -> [w379 _ _]
                tunnel: w359 -> [_ _ w409]
                frame #0 {
                  n95 = Index Array(array=w390, index=w389) -> (element=w387:dbl)
                  n96 = Index Array(array=w392, index=w389) -> ()  [unwired: 1 out]
                  n97 = Index Array(array=w391, index=w389) -> ()  [unwired: 1 out]
                  n98 = Index Array(array=w394, index=w389) -> (element=w393:string)
                  n99 = Number To Fractional String(use system decimal point (T)=FALSE ("Systemdezimalzeichen verwenden (T)"), number=w382) -> (F-format string=w381:string)  [unwired: 2 in]
                  n100 = Number To Fractional String(use system decimal point (T)=FALSE ("Systemdezimalzeichen verwenden (T)"), number=w387) -> (F-format string=w385:string)  [unwired: 2 in]
                  n101 = call "Traegergas aus Verduennungsgas.vi"("Verdünnungsgas"=w379) -> ("Trägergas"=w402:T3)  [unwired: 10 in]
                  n102 = call "GD_MG_MagicFormula_OnOff.vi"("Aktion"=enum16{"lesen", "schreiben", "init"}."lesen") -> ("MG_use_magic_formula"=w386:bool)  [unwired: 8 in, 1 out]
                  n103 = Select(t=w381, s=w386, f=w385) -> (s? t:f=w384:string)
                  n104 = Equal?(x=w402, y=T3 "O2") -> (x = y?=w404:bool)
                  n105 = Select(t="SL" ("Formel"), s=w404, f=w402) -> (s? t:f=w401:T3)
                  n106 = Build Array(w401, w393, w384) -> (w400:T3[])
                  n107 = call "AK Komm.vi"("Aktionen"=Aktionen_AK_Komm."EGAK", "Daten"=w400) -> ("Empfangsdaten"=w398:string[], "Error"=w397:T33, "Status"=w399:string, "Störung Kommunikation"=w396:bool)  [unwired: 3 in, 3 out]
                  n108 = call "Map GD Errors.vi"("Error"=w397, "Störung Kommunikation"=w396) -> ("LIN Errors-Cluster (Ausgang)"=w395:T29)  [unwired: 8 in, 1 out]
                }
                frame #1 {
                  n109 = call "AK Komm.vi"("Aktionen"=Aktionen_AK_Komm."AGAK") -> ("Empfangsdaten"=w407:string[])  [unwired: 4 in, 6 out]
                }
                frame #2 {
                }
              }
            }
            frame 3 {
              # "Horiba GDC"
              n110 = stacked-sequence {
                tunnel: w428 -> [w447 _ _]
                tunnel: w427 -> [w437 _ _]
                tunnel: w426 -> [w436 _ _]
                tunnel: w425 -> [_ _ _]
                tunnel: w424 -> [w446 _ _]
                tunnel: w423 -> [_ _ _]
                tunnel: [_ _ w483] -> w411
                tunnel: [_ w479 _] -> w422
                tunnel: [_ w479 _] -> w421
                tunnel: [w445 _ _] -> w420
                tunnel: [w444 _ _] -> w419
                tunnel: w418 -> [w440 _ _]
                tunnel: w417 -> [w438 _ _]
                tunnel: w416 -> [w434 _ _]
                tunnel: w415 -> [w432 _ _]
                tunnel: w414 -> [_ _ _]
                tunnel: w413 -> [_ _ _]
                tunnel: w412 -> [_ _ _]
                tunnel: w410 -> [_ _ w483]
                frame #0 {
                  n111 = Index Array(array=w436, index=w434) -> (element=w431:dbl)
                  n112 = Index Array(array=w437, index=w434) -> ()  [unwired: 1 out]
                  n113 = Index Array(array=w438, index=w434) -> (element=w435:string)
                  n114 = Index Array(array=w440, index=w434) -> (element=w439:string)
                  n115 = call "GD_MG_MagicFormula_OnOff.vi"("Aktion"=enum16{"lesen", "schreiben", "init"}."lesen") -> ("MG_use_magic_formula"=w433:bool)  [unwired: 8 in, 1 out]
                  n116 = Number To Fractional String(number=w447, width (-)=i16 3 ("Breite (-)"), precision (6)=i16 0 ("Genauigkeit (6)")) -> (F-format string=w448:string)  [unwired: 1 in]
                  n117 = Select(t=w432, s=w433, f=w431) -> (s? t:f=w430:dbl)
                  n118 = case shown="\"ppm\", Standard" w435 {
                    tunnel: [i16 1 ("Genauigkeit (6)") i16 3 ("Genauigkeit (6)")] -> w458
                    tunnel: w430 -> [w468 w473]
                    tunnel: [w468 w472] -> w459
                    tunnel: ["ppm" "%"] -> w456
                    tunnel: w431 -> [_ w470]
                    frame "ppm", Default {
                      # "ppm"
                    }
                    frame "%" {
                      n119 = disable-structure shown="Aktiviert" {
                        disable-tunnel: w473 -> [_ w478]
                        disable-tunnel: [w477 w478] -> w472
                        disable-tunnel: w470 -> [w475 _]
                        frame Disabled {
                          # "%"
                          n120 = Multiply(x=w475, y=T5 10000.0) -> (x*y=w477:dbl)
                        }
                        frame Enabled {
                        }
                      }
                    }
                  }
                  n121 = Number To Decimal String(number=w446) -> (decimal integer string=w454:string)  [unwired: 1 in]
                  n122 = case shown="\"CH4\"" w439 {
                    tunnel: ["2" "3" "4" "5" "7" "1" "1"] -> w449
                    frame "CO2" {
                    }
                    frame "O2" {
                    }
                    frame "CH4" {
                    }
                    frame "C3H8" {
                    }
                    frame "NO" {
                    }
                    frame "0", Default {
                    }
                    frame "CO" {
                    }
                  }
                  n123 = Number To Fractional String(use system decimal point (T)=FALSE ("Systemdezimalzeichen verwenden (T)"), number=w459, precision (6)=w458) -> (F-format string=w455:string)  [unwired: 1 in]
                  n124 = Build Array(w449, w454, w448, w455, w456) -> (w452:string[])
                  n125 = call "GDC Kom.vi"("Befehl"=Aktion_Befehl."GD parameter", "Daten"=w452) -> ("Status (alarm)"=w441:bool, "Fehler"=w442:bool, "Status"=w445:string)  [unwired: 3 in, 4 out]
                  n126 = call "Map GD Errors.vi"("Störung Gasteiler"=w441, "Error"=T33 {"Pressure carrier gas"=FALSE, "Pressure diluted gas"=FALSE, "Outlet Pressure"=FALSE, "SNOX before SAIR"=FALSE}, "Störung Kommunikation"=w442) -> ("LIN Errors-Cluster (Ausgang)"=w444:T29)  [unwired: 7 in, 1 out]
                }
                frame #1 {
                  n127 = call "GDC Kom.vi"("Befehl"=Aktion_Befehl."Info") -> ("Gas"=w481:string[], "Konzentration 2"=w480:string)  [unwired: 4 in, 5 out]
                  n128 = Build Array (concatenate)(w481, w480) -> (w479:string[])
                }
                frame #2 {
                  n129 = call "GDC Kom.vi"("Befehl"=Aktion_Befehl."Standby") -> ()  [unwired: 4 in, 7 out]
                }
              }
            }
            frame 4 {
              # "HovaCAL #Option10xSpanAuto\nwird in HavaCAL Komm gemacht,\naber damit man es sieht ?"
            }
            frame 5 {
              # "Horiba 710 c ... manuell !"
            }
          }
          n130 = call "GD TimeStamp.vi"() -> ("date/time string"=w137:string)  [unwired: 10 in, 1 out]
          n131 = Bundle By Name(cluster=T28 {"Wobei"="", "Status"="", "Errors"={"Störung Kommunikation"=FALSE, "Pressure carrier gas"=FALSE, "Pressure diluted gas"=FALSE, "Outlet Pressure"=FALSE, "SNOX before SAIR"=FALSE, "Störung Gasteiler"=FALSE}, "Empfangsdaten"=[], "Zeitstempel"=""} ("GD Info-Cluster"), "Zeitstempel"=w137, "Wobei"="GD get Table of Points" ("Status"), "Status"=w155, "Errors"=w154, "Empfangsdaten"=w153) -> (w152:T28)
          n132 = case shown="True" w151 {
            tunnel: w152 -> [_ w492]
            tunnel: w150 -> [_ w490]
            frame False {
            }
            frame True {
              n133 = call "Status mit GD Info aktualisieren.vi"("show Status even if no Error"=TRUE, "Sprachliste"=w490, "GD Info-Cluster in"=w492) -> ("Status out"=w489:string)  [unwired: 7 in, 1 out]
              n134 = local write "Status out"(w489) -> ()
            }
          }
          n135 = call "FGV GD Errors sammeln.vi"("Aktion"=Aktion_FGV_GD_Errors_sammeln."GD Infos sammeln", "GD Info-Cluster in"=w152) -> ()  [unwired: 7 in, 3 out]
        }
        frame True {
          # "Wenn 0 (----) kommt dann nicht abfragen"
        }
      }
    }
    frame True {
      # "Stufentabelle neu abfragen"
      n136 = case shown="False" w511 {
        tunnel: w515 -> [w556 _]
        tunnel: w517 -> [w555 _]
        tunnel: w516 -> [w554 _]
        tunnel: w514 -> [w553 _]
        tunnel: w522 -> [w552 _]
        tunnel: w521 -> [w551 _]
        tunnel: w520 -> [w550 _]
        tunnel: w519 -> [w546 w1138]
        tunnel: [w549 w1138] -> w518
        tunnel: [w548 w1137] -> w513
        tunnel: [w547 _] -> w512
        tunnel: w510 -> [w538 _]
        tunnel: w509 -> [w537 _]
        tunnel: w508 -> [w536 _]
        tunnel: w507 -> [w535 _]
        tunnel: w506 -> [w534 _]
        tunnel: w505 -> [w533 _]
        tunnel: w504 -> [w532 _]
        tunnel: w503 -> [w531 _]
        tunnel: w502 -> [w530 _]
        tunnel: w501 -> [w529 _]
        tunnel: w500 -> [w528 _]
        tunnel: w499 -> [w527 _]
        tunnel: w498 -> [w526 _]
        tunnel: w497 -> [w525 _]
        tunnel: w496 -> [w524 _]
        tunnel: w495 -> [_ w1137]
        frame False {
          # "#GD_Error_TimeStamp"
          n137 = case shown="0, Standard" w556 {
            tunnel: w555 -> [w580 w802 w871 w946 _ _]
            tunnel: w554 -> [w579 w801 w870 w945 _ _]
            tunnel: w553 -> [w578 w800 w859 w947 w1074 _]
            tunnel: w552 -> [w577 w798 w853 w943 _ _]
            tunnel: w551 -> [w576 w799 w869 w944 w1073 _]
            tunnel: w550 -> [w575 w797 w868 w942 w1072 w1101]
            tunnel: [w574 w785 w854 w930 w1065 w1096] -> w549
            tunnel: [w573 w796 w866 w941 _ _] -> w548
            tunnel: [w572 _ w867 w940 _ _] -> w547
            tunnel: w546 -> [_ _ _ _ _ _]
            tunnel: [w571 w795 w865 w939 _ _] -> w542
            tunnel: [w570 w793 w863 w938 _ _] -> w541
            tunnel: [w564 w794 w864 _ _ _] -> w540
            tunnel: w536 -> [w569 w791 w862 w937 _ _]
            tunnel: w535 -> [w568 w792 w861 w936 w1066 w1099]
            tunnel: w534 -> [_ _ _ _ w1071 _]
            tunnel: w533 -> [w567 _ _ _ _ _]
            tunnel: w532 -> [w566 _ _ _ _ _]
            tunnel: w531 -> [w565 _ _ _ _ _]
            tunnel: w530 -> [w563 w786 w858 w934 w1056 w1091]
            tunnel: w529 -> [w562 w790 w860 w935 w1059 w1089]
            tunnel: w528 -> [w561 w788 w856 w931 w1060 w1090]
            tunnel: w527 -> [w560 w789 w857 w933 w1068 w1100]
            tunnel: w526 -> [w559 w787 w855 w932 w1067 w1098]
            tunnel: w525 -> [w558 _ _ _ _ _]
            tunnel: w524 -> [w557 _ _ _ _ _]
            frame 0, Default {
              # "LCD-Touch Display"
              n138 = case shown="True" w567 {
                tunnel: w580 -> [w602 w733]
                tunnel: w579 -> [w600 w732]
                tunnel: w578 -> [w592 w731]
                tunnel: w577 -> [w597 w730]
                tunnel: w576 -> [w599 w729]
                tunnel: w575 -> [w591 w728]
                tunnel: [w587 w727] -> w574
                tunnel: [w590 w726] -> w573
                tunnel: [w589 w725] -> w572
                tunnel: [w595 w724] -> w571
                tunnel: [w594 w722] -> w570
                tunnel: w569 -> [w588 w721]
                tunnel: w568 -> [w601 w720]
                tunnel: w566 -> [w598 _]
                tunnel: w565 -> [w596 _]
                tunnel: [w593 w723] -> w564
                tunnel: w563 -> [_ w716]
                tunnel: w562 -> [w583 w719]
                tunnel: w561 -> [w584 w715]
                tunnel: w560 -> [w586 w718]
                tunnel: w559 -> [w585 w717]
                tunnel: w558 -> [w582 _]
                tunnel: w557 -> [w581 _]
                frame False {
                  n139 = stacked-sequence {
                    seq-local: [w603 _ _ _] -> [_ w617 _ _]
                    seq-local: [_ w616 _ _] -> [_ _ w638 _]
                    seq-local: [_ _ w637 _] -> [_ _ _ _]
                    tunnel: w601 -> [_ _ _ w661]
                    tunnel: w600 -> [_ _ _ _]
                    tunnel: [_ w631 _ _] -> w595
                    tunnel: [_ w614 _ _] -> w593
                    tunnel: [_ w629 _ _] -> w594
                    tunnel: w598 -> [w612 w627 w647 _]
                    tunnel: w596 -> [_ w626 _ _]
                    tunnel: [_ w618 _ _] -> _
                    tunnel: w602 -> [_ _ _ _]
                    tunnel: w599 -> [_ _ _ w668]
                    tunnel: w597 -> [_ w615 _ _]
                    tunnel: w592 -> [_ _ _ w670]
                    tunnel: w591 -> [_ _ _ w669]
                    tunnel: [_ w614 _ _] -> w590
                    tunnel: [_ _ w636 _] -> w589
                    tunnel: w588 -> [_ _ _ w664]
                    tunnel: [_ _ _ w662] -> w587
                    tunnel: w586 -> [_ _ _ w652]
                    tunnel: w585 -> [_ _ _ w651]
                    tunnel: w584 -> [_ _ _ w658]
                    tunnel: w583 -> [_ _ _ w656]
                    tunnel: w582 -> [_ _ w635 w655]
                    tunnel: w581 -> [_ _ _ w654]
                    frame #0 {
                      # "Delete Cylinder if already exists, ignore DF Error if not yet\n\nIf SE or ???? retun for command then old SW version ..."
                      n140 = Build Array(w612) -> (w611:string[])
                      n141 = call "AK Komm.vi"("Aktionen"=Aktionen_AK_Komm."DCYL", "Daten"=w611) -> ("Empfangsdaten"=w610:string[])  [unwired: 3 in, 6 out]
                      n142 = Index Array(array=w610) -> (element #1=w609:string, element #2=w606:string)  [unwired: 2 in]
                      n143 = Equal?(x=w606, y="SE") -> (x = y?=w604:bool)
                      n144 = Not Equal?(x=w609, y="DCAL") -> (x != y?=w607:bool)
                      n145 = Or(x=w607, y=w604) -> (x .or. y?=w603:bool)
                    }
                    frame #1 {
                      # "Create new Cylinder \nIf DF Formula of Gas wrong ... or use AGAT to get gaslist und search for Formula if exists ?\nIf SE or ???? retun for command then old SW version ..."
                      n146 = call "Traegergas aus Verduennungsgas.vi"("Verdünnungsgas"=w615) -> ("Trägergas"=w633:T3)  [unwired: 10 in]
                      n147 = Build Array (concatenate)(w627, w633, w626) -> (w632:T3[])
                      n148 = call "AK Komm.vi"("Aktionen"=Aktionen_AK_Komm."SCYL", "Daten"=w632) -> ("Empfangsdaten"=w614:string[], "Error"=w630:T33, "Status"=w631:string, "Störung Kommunikation"=w628:bool)  [unwired: 3 in, 3 out]
                      n149 = Index Array(array=w614) -> (element #1=w625:string, element #2=w622:string)  [unwired: 2 in]
                      n150 = call "Map GD Errors.vi"("Error"=w630, "Störung Kommunikation"=w628) -> ("LIN Errors-Cluster (Ausgang)"=w629:T29)  [unwired: 8 in, 1 out]
                      n151 = Equal?(x=w622, y="SE") -> (x = y?=w619:bool)
                      n152 = Equal?(x=w622, y="DF") -> (x = y?=w618:bool)
                      n153 = Not Equal?(x=w625, y="SCYL") -> (x != y?=w620:bool)
                      n154 = Compound Arithmetic op=OR ("Mehrfacharithmetik")(w617, w620, w619) -> (w616:bool)
                    }
                    frame #2 {
                      # "use the defined Cylinder"
                      n155 = Build Array(w647, "DIL", w635) -> (w648:string[])
                      n156 = call "AK Komm.vi"("Aktionen"=Aktionen_AK_Komm."CCYL", "Daten"=w648) -> ("Empfangsdaten"=w636:string[])  [unwired: 3 in, 6 out]
                      n157 = Index Array(array=w636) -> (element #1=w645:string, element #2=w642:string)  [unwired: 2 in]
                      n158 = Equal?(x=w642, y="SE") -> (x = y?=w639:bool)
                      n159 = Equal?(x=w642, y="DF") -> ()  [unwired: 1 out]
                      n160 = Not Equal?(x=w645, y="CCYL") -> (x != y?=w640:bool)
                      n161 = Compound Arithmetic op=OR ("Mehrfacharithmetik")(w638, w640, w639) -> (w637:bool)
                    }
                    frame #3 {
                      # "Get a point for all components in cylinder ...\n\nDRGV 0 N2 TestUnit 9 CO2 1.729 N2 9.983E+08 NO2 1.729 O2 1.642E+06"
                      n162 = Index Array(array=w658, index=w656) -> (element=w653:dbl)
                      n163 = call "Stufen gleichmäßig aufteilen.vi"("Punkte umkehren"=w669, "Stufen"=w668, "Anzahl"=w670) -> ("Stufen"=w667:u16[])  [unwired: 8 in]
                      n164 = Number To Decimal String(number=w667) -> (decimal integer string=w663:string[])  [unwired: 1 in]
                      n165 = for {
                        tunnel: [w708] -> w666
                        tunnel: [w707] -> w665 mode=indexing
                        tunnel: w663 -> [w706] mode=indexing
                        tunnel: w655 -> [w705]
                        tunnel: w654 -> [w704]
                        n166 = Build Array(w704, w705, w706) -> (w713:string[])
                        n167 = call "AK Komm.vi"("Aktionen"=Aktionen_AK_Komm."DRGV", "Daten"=w713) -> ("Empfangsdaten"=w712:string[])  [unwired: 3 in, 6 out]
                        n168 = Delete From Array(array=w712, length=4 ("Länge"), index=0 ("Index")) -> (array with subset deleted=w709:string[])  [unwired: 1 out]
                        n169 = call "Gase und Konzentrationen splitten.vi"("Empfangsdaten (Eingang)"=w709) -> ("Konzentrationen"=w707:string[], "Gase"=w708:string[])  [unwired: 9 in]
                      }
                      n170 = Empty Array?(array=w651) -> (empty?=w650:bool)
                      n171 = call "Konzentrationn in Reihenfolge bringen.vi"("Gas Namen"=w664, "Konzentrationen"=w665, "Gase"=w666) -> ("Stufen ja Gas"=w657:string[][])  [unwired: 8 in]
                      n172 = for {
                        tunnel: w661 -> [w699] mode=indexing
                        tunnel: w657 -> [w698] mode=indexing
                        tunnel: [w697] -> w659 mode=indexing
                        n173 = for {
                          tunnel: w699 -> [w703]
                          tunnel: w698 -> [w701] mode=indexing
                          tunnel: [w702] -> w697 mode=indexing
                          n174 = call "ppm wieder in Prozent umrechnen.vi"("LNI_ppb"=TRUE, "Einheit"=w703, "Werteingang"=w701) -> ("Wertausgang"=w702:string)  [unwired: 8 in]
                        }
                      }
                      n175 = case shown="False" w650 {
                        tunnel: [w679 w692] -> w660
                        tunnel: w659 -> [w678 w692]
                        tunnel: w657 -> [w677 _]
                        tunnel: w656 -> [w676 _]
                        tunnel: w653 -> [w674 _]
                        tunnel: w652 -> [w673 _]
                        tunnel: w651 -> [w672 _]
                        frame False {
                          n176 = Index Array(array=w677, index (row)=w676) -> (element=w675:string[])  [unwired: 1 in]
                          n177 = for {
                            tunnel: w675 -> [w684]
                            tunnel: w674 -> [w683]
                            tunnel: w673 -> [w682] mode=indexing
                            tunnel: w672 -> [w681] mode=indexing
                            tunnel: [w680] -> w671
                            n178 = for {
                              tunnel: w682 -> [w690]
                              tunnel: w681 -> [w689]
                              tunnel: w684 -> [w686] mode=indexing
                              tunnel: w683 -> [w688]
                              tunnel: [w687] -> w680 mode=indexing
                              n179 = call "ppb in ppm.vi"("Werteingang"=w686) -> ("Wertausgang"=w685:string)  [unwired: 9 in]
                              n180 = call "Konzentration der einzelnen Komponente umrechnen.vi"("Teilkonzentration"=w690, "Gesamtkonzentration"=w688, "Werteingang"=w685) -> ("Wertausgang"=w691:string)  [unwired: 8 in]
                              n181 = call "ppm wieder in Prozent umrechnen.vi"("Einheit"=w689, "Werteingang"=w691) -> ("Wertausgang"=w687:string)  [unwired: 9 in]
                            }
                          }
                          n182 = Build Array (concatenate)(w671, w678) -> (w679:string[][])
                        }
                        frame True {
                        }
                      }
                      n183 = for {
                        tunnel: w663 -> [w695]
                        tunnel: w660 -> [w694] mode=indexing
                        tunnel: [w693] -> w662 mode=indexing
                        n184 = Build Array(w695, w694) -> (w696:string[][])
                        n185 = Transpose 2D Array(2D array=w696) -> (transposed array=w693:string[][])
                      }
                    }
                  }
                }
                frame True {
                  n186 = stacked-sequence {
                    tunnel: w733 -> [w746 _ _]
                    tunnel: w732 -> [_ _ _]
                    tunnel: w731 -> [_ _ w777]
                    tunnel: w730 -> [w756 _ _]
                    tunnel: w729 -> [_ _ w776]
                    tunnel: w728 -> [_ _ w775]
                    tunnel: [_ _ w772] -> w727
                    tunnel: [w754 _ _] -> w726
                    tunnel: [_ w758 _] -> w725
                    tunnel: [w753 _ _] -> w724
                    tunnel: [w752 _ _] -> w723
                    tunnel: [w750 _ _] -> w722
                    tunnel: w721 -> [w748 _ _]
                    tunnel: w720 -> [w745 _ w771]
                    tunnel: w719 -> [w744 _ w761]
                    tunnel: w718 -> [_ _ w774]
                    tunnel: w717 -> [_ _ w773]
                    tunnel: w716 -> [w742 _ w763]
                    tunnel: w715 -> [w738 _ w764]
                    frame #0 {
                      n187 = Index Array(array=w738, index=w744) -> (element=w736:dbl)
                      n188 = Index Array(array=w746, index=w744) -> ()  [unwired: 1 out]
                      n189 = Index Array(array=w745, index=w744) -> ()  [unwired: 1 out]
                      n190 = Index Array(array=w748, index=w744) -> (element=w747:string)
                      n191 = Number To Fractional String(use system decimal point (T)=FALSE ("Systemdezimalzeichen verwenden (T)"), number=w742) -> (F-format string=w740:string)  [unwired: 2 in]
                      n192 = Number To Fractional String(use system decimal point (T)=FALSE ("Systemdezimalzeichen verwenden (T)"), number=w736) -> (F-format string=w735:string)  [unwired: 2 in]
                      n193 = call "Traegergas aus Verduennungsgas.vi"("Verdünnungsgas"=w756) -> ("Trägergas"=w755:T3)  [unwired: 10 in]
                      n194 = call "GD_MG_MagicFormula_OnOff.vi"("Aktion"=enum16{"lesen", "schreiben", "init"}."lesen") -> ("MG_use_magic_formula"=w741:bool)  [unwired: 8 in, 1 out]
                      n195 = Select(t=w740, s=w741, f=w735) -> (s? t:f=w739:string)
                      n196 = Build Array(w755, w747, w739) -> (w754:T3[])
                      n197 = call "AK Komm.vi"("Aktionen"=Aktionen_AK_Komm."EGAK", "Daten"=w754) -> ("Empfangsdaten"=w752:string[], "Error"=w751:T33, "Status"=w753:string, "Störung Kommunikation"=w749:bool)  [unwired: 3 in, 3 out]
                      n198 = call "Map GD Errors.vi"("Error"=w751, "Störung Kommunikation"=w749) -> ("LIN Errors-Cluster (Ausgang)"=w750:T29)  [unwired: 8 in, 1 out]
                    }
                    frame #1 {
                      n199 = call "AK Komm.vi"("Aktionen"=Aktionen_AK_Komm."AGAK") -> ("Empfangsdaten"=w758:string[])  [unwired: 4 in, 6 out]
                    }
                    frame #2 {
                      n200 = Index Array(array=w764, index=w761) -> (element=w765:dbl)
                      n201 = call "Stufen gleichmäßig aufteilen.vi"("Punkte umkehren"=w775, "Stufen"=w776, "Anzahl"=w777) -> ("Stufen"=w778:u16[])  [unwired: 8 in]
                      n202 = Build Array (concatenate)(w774, w764) -> (w770:dbl[])
                      n203 = Number To Decimal String(number=w778) -> (decimal integer string=w768:string[])  [unwired: 1 in]
                      n204 = call "GD_MG_MagicFormula_OnOff.vi"("Aktion"=enum16{"lesen", "schreiben", "init"}."lesen") -> ("MG_use_magic_formula"=w766:bool)  [unwired: 8 in, 1 out]
                      n205 = Build Array (concatenate)(w773, w771) -> (w769:string[])
                      n206 = Select(t=w763, s=w766, f=w765) -> (s? t:f=w762:dbl)
                      n207 = for {
                        tunnel: w768 -> [w783] mode=indexing
                        tunnel: [w779] -> w767 mode=indexing
                        stop <- w780 stop-if-true
                        n208 = Build Array(w783) -> (w782:string[])
                        n209 = call "AK Komm.vi"("Aktionen"=Aktionen_AK_Komm."AKAK", "Daten"=w782) -> ("Empfangsdaten"=w781:string[], "Störung Kommunikation"=w780:bool)  [unwired: 3 in, 5 out]
                        n210 = Index Array(array=w781) -> (element=w779:string)  [unwired: 1 in]
                      }
                      n211 = call "GD_GesamtKonz_back_calc.vi"("Gesamtkonzentration"=w762, "Einheiten"=w769, "Konzentration der Komponenten"=w770, "Stufen"=w767, "Punkte (Eingang)"=w768) -> ("Stufentabellen (Ausgang)"=w772:string[][][])  [unwired: 5 in, 1 out]
                    }
                  }
                }
              }
            }
            frame 1 {
              # "Analog-Display"
              n212 = stacked-sequence {
                tunnel: w802 -> [_ _]
                tunnel: w801 -> [_ _]
                tunnel: w800 -> [_ w842]
                tunnel: w799 -> [_ w841]
                tunnel: w798 -> [w823 _]
                tunnel: w797 -> [_ w840]
                tunnel: [_ w836] -> w785
                tunnel: [w821 _] -> w796
                tunnel: [w820 _] -> w795
                tunnel: [w817 _] -> w793
                tunnel: [w819 _] -> w794
                tunnel: w792 -> [_ w837]
                tunnel: w791 -> [w815 _]
                tunnel: w790 -> [w813 w827]
                tunnel: w789 -> [_ w839]
                tunnel: w788 -> [w807 w828]
                tunnel: w787 -> [_ w838]
                tunnel: w786 -> [w811 w829]
                frame #0 {
                  n213 = Index Array(array=w807, index=w813) -> (element=w806:dbl)
                  n214 = Index Array(array=w815, index=w813) -> (element=w814:string)
                  n215 = Number To Fractional String(use system decimal point (T)=FALSE ("Systemdezimalzeichen verwenden (T)"), number=w811) -> (F-format string=w809:string)  [unwired: 2 in]
                  n216 = Number To Fractional String(use system decimal point (T)=FALSE ("Systemdezimalzeichen verwenden (T)"), number=w806) -> (F-format string=w804:string)  [unwired: 2 in]
                  n217 = call "Traegergas aus Verduennungsgas.vi"("Verdünnungsgas"=w823) -> ("Trägergas"=w822:T3)  [unwired: 10 in]
                  n218 = call "GD_MG_MagicFormula_OnOff.vi"("Aktion"=enum16{"lesen", "schreiben", "init"}."lesen") -> ("MG_use_magic_formula"=w810:bool)  [unwired: 8 in, 1 out]
                  n219 = Select(t=w809, s=w810, f=w804) -> (s? t:f=w808:string)
                  n220 = Build Array(w822, w814, w808) -> (w821:T3[])
                  n221 = call "AK Komm_ALT.vi"("Aktionen_ALT"=Aktionen_AK_Komm_ALT."EGAK", "Daten"=w821) -> ("Empfangsdaten"=w819:string[], "Error"=w818:T33, "Status"=w820:string, "Störung Kommunikation"=w816:bool)  [unwired: 5 in, 1 out]
                  n222 = call "Map GD Errors.vi"("Error"=w818, "Störung Kommunikation"=w816) -> ("LIN Errors-Cluster (Ausgang)"=w817:T29)  [unwired: 8 in, 1 out]
                }
                frame #1 {
                  n223 = call "AK Komm_ALT.vi"("Aktionen_ALT"=Aktionen_AK_Komm_ALT."AGAK") -> ("Empfangsdaten"=w848:string[])  [unwired: 6 in, 4 out]
                  n224 = Index Array(array=w828, index=w827) -> (element=w826:dbl)
                  n225 = call "Stufen gleichmäßig aufteilen.vi"("Punkte umkehren"=w840, "Stufen"=w841, "Anzahl"=w842) -> ("Stufen"=w850:u16[])  [unwired: 8 in]
                  n226 = Build Array (concatenate)(w839, w828) -> (w833:dbl[])
                  n227 = call "AK Komm_ALT.vi"("Aktionen_ALT"=Aktionen_AK_Komm_ALT."ALST") -> ("Empfangsdaten"=w851:string[])  [unwired: 6 in, 4 out]
                  n228 = Index Array(array=w848, index=2 ("Index")) -> (element=w845:string)
                  n229 = Number To Decimal String(number=w850) -> (decimal integer string=w835:string[])  [unwired: 1 in]
                  n230 = Build Array (concatenate)(w838, w837) -> (w832:string[])
                  n231 = Fract/Exp String To Number(use system decimal point (T)=TRUE ("Systemdezimalzeichen verwenden (T)"), string=w845, default (0 dbl)=sgl 0.0 ("Standard (0 DBL)")) -> (number=w844:sgl)  [unwired: 1 in, 1 out]
                  n232 = call "GD_MG_MagicFormula_OnOff.vi"("Aktion"=enum16{"lesen", "schreiben", "init"}."lesen") -> ("MG_use_magic_formula"=w831:bool)  [unwired: 8 in, 1 out]
                  n233 = call "Stufen berechnen.vi"("Empfangsdaten"=w851, "Konzentration"=w844, "Stufen"=w850) -> ("Stufen Tabelle"=w834:string[])  [unwired: 7 in, 1 out]
                  n234 = Select(t=w829, s=w831, f=w826) -> (s? t:f=w830:dbl)
                  n235 = call "GD_GesamtKonz_back_calc.vi"("Gesamtkonzentration"=w830, "Einheiten"=w832, "Konzentration der Komponenten"=w833, "Stufen"=w834, "Punkte (Eingang)"=w835) -> ("Stufentabellen (Ausgang)"=w836:string[][][])  [unwired: 5 in, 1 out]
                }
              }
            }
            frame 2 {
              # "AVL GDU"
              n236 = stacked-sequence {
                tunnel: w859 -> [_ _ w919]
                tunnel: w871 -> [w885 _ _]
                tunnel: w870 -> [_ _ _]
                tunnel: w869 -> [_ _ w918]
                tunnel: w868 -> [_ _ w917]
                tunnel: [_ w900 _] -> w867
                tunnel: [_ _ w913] -> w854
                tunnel: [w893 _ _] -> w866
                tunnel: [w892 _ _] -> w865
                tunnel: [w891 _ _] -> w864
                tunnel: [w888 _ _] -> w863
                tunnel: w862 -> [w887 _ _]
                tunnel: w861 -> [w884 _ w914]
                tunnel: w860 -> [w882 _ w903]
                tunnel: w858 -> [w875 _ w904]
                tunnel: w857 -> [_ _ w916]
                tunnel: w856 -> [w883 _ w906]
                tunnel: w855 -> [_ _ w915]
                tunnel: w853 -> [w872 _ _]
                frame #0 {
                  n237 = Index Array(array=w883, index=w882) -> (element=w880:dbl)
                  n238 = Index Array(array=w885, index=w882) -> ()  [unwired: 1 out]
                  n239 = Index Array(array=w884, index=w882) -> ()  [unwired: 1 out]
                  n240 = Index Array(array=w887, index=w882) -> (element=w886:string)
                  n241 = Number To Fractional String(use system decimal point (T)=FALSE ("Systemdezimalzeichen verwenden (T)"), number=w875) -> (F-format string=w874:string)  [unwired: 2 in]
                  n242 = Number To Fractional String(use system decimal point (T)=FALSE ("Systemdezimalzeichen verwenden (T)"), number=w880) -> (F-format string=w878:string)  [unwired: 2 in]
                  n243 = call "Traegergas aus Verduennungsgas.vi"("Verdünnungsgas"=w872) -> ("Trägergas"=w895:T3)  [unwired: 10 in]
                  n244 = call "GD_MG_MagicFormula_OnOff.vi"("Aktion"=enum16{"lesen", "schreiben", "init"}."lesen") -> ("MG_use_magic_formula"=w879:bool)  [unwired: 8 in, 1 out]
                  n245 = Select(t=w874, s=w879, f=w878) -> (s? t:f=w877:string)
                  n246 = Equal?(x=w895, y=T3 "O2") -> (x = y?=w897:bool)
                  n247 = Select(t="SL" ("Formel"), s=w897, f=w895) -> (s? t:f=w894:T3)
                  n248 = Build Array(w894, w886, w877) -> (w893:T3[])
                  n249 = call "AK Komm.vi"("Aktionen"=Aktionen_AK_Komm."EGAK", "Daten"=w893) -> ("Empfangsdaten"=w891:string[], "Error"=w890:T33, "Status"=w892:string, "Störung Kommunikation"=w889:bool)  [unwired: 3 in, 3 out]
                  n250 = call "Map GD Errors.vi"("Error"=w890, "Störung Kommunikation"=w889) -> ("LIN Errors-Cluster (Ausgang)"=w888:T29)  [unwired: 8 in, 1 out]
                }
                frame #1 {
                  n251 = call "AK Komm.vi"("Aktionen"=Aktionen_AK_Komm."AGAK") -> ("Empfangsdaten"=w900:string[])  [unwired: 4 in, 6 out]
                }
                frame #2 {
                  n252 = call "Stufen gleichmäßig aufteilen.vi"("Punkte umkehren"=w917, "Stufen"=w918, "Anzahl"=w919) -> ("Stufen"=w920:u16[])  [unwired: 8 in]
                  n253 = Index Array(array=w906, index=w903) -> (element=w907:dbl)
                  n254 = Number To Decimal String(number=w920) -> (decimal integer string=w912:string[])  [unwired: 1 in]
                  n255 = Build Array (concatenate)(w916, w906) -> (w910:dbl[])
                  n256 = Build Array (concatenate)(w915, w914) -> (w909:string[])
                  n257 = call "GD_MG_MagicFormula_OnOff.vi"("Aktion"=enum16{"lesen", "schreiben", "init"}."lesen") -> ("MG_use_magic_formula"=w908:bool)  [unwired: 8 in, 1 out]
                  n258 = Select(t=w904, s=w908, f=w907) -> (s? t:f=w905:dbl)
                  n259 = for {
                    tunnel: w912 -> [w928] mode=indexing
                    tunnel: [w923] -> w911 mode=indexing
                    tunnel: w905 -> [w922]
                    stop <- w925 stop-if-true
                    n260 = Build Array(w928) -> (w927:string[])
                    n261 = call "AK Komm.vi"("Aktionen"=Aktionen_AK_Komm."ALST", "Daten"=w927) -> ("Empfangsdaten"=w926:string[], "Störung Kommunikation"=w925:bool)  [unwired: 3 in, 5 out]
                    n262 = Index Array(array=w926, index=1 ("Index")) -> (element=w921:string)
                    n263 = call "AVL GNU umrechnen ALST.vi"("Konzentration"=w922, "Teilerstufe in%"=w921) -> ("Konzentration"=w923:string)  [unwired: 9 in]
                  }
                  n264 = call "GD_GesamtKonz_back_calc.vi"("Gesamtkonzentration"=w905, "Einheiten"=w909, "Konzentration der Komponenten"=w910, "Stufen"=w911, "Punkte (Eingang)"=w912) -> ("Stufentabellen (Ausgang)"=w913:string[][][])  [unwired: 5 in, 1 out]
                }
              }
            }
            frame 3 {
              # "Horiba GDC"
              n265 = stacked-sequence {
                tunnel: w947 -> [w966 _ w1020 _]
                tunnel: w946 -> [w956 _ _ _]
                tunnel: w945 -> [w955 _ _ _]
                tunnel: w944 -> [_ _ w1019 _]
                tunnel: w943 -> [w965 _ _ _]
                tunnel: w942 -> [_ _ w1018 _]
                tunnel: [_ _ w1014 _] -> w930
                tunnel: [_ w998 _ _] -> w941
                tunnel: [_ w998 _ _] -> w940
                tunnel: [w964 _ _ _] -> w939
                tunnel: [w963 _ _ _] -> w938
                tunnel: w937 -> [w959 _ _ _]
                tunnel: w936 -> [w957 _ w1015 _]
                tunnel: w935 -> [w953 _ w1005 _]
                tunnel: w934 -> [w951 _ w1004 _]
                tunnel: w933 -> [_ _ w1017 _]
                tunnel: w932 -> [_ _ w1016 _]
                tunnel: w931 -> [_ _ w1006 _]
                frame #0 {
                  n266 = Index Array(array=w955, index=w953) -> (element=w950:dbl)
                  n267 = Index Array(array=w956, index=w953) -> ()  [unwired: 1 out]
                  n268 = Index Array(array=w957, index=w953) -> (element=w954:string)
                  n269 = Index Array(array=w959, index=w953) -> (element=w958:string)
                  n270 = call "GD_MG_MagicFormula_OnOff.vi"("Aktion"=enum16{"lesen", "schreiben", "init"}."lesen") -> ("MG_use_magic_formula"=w952:bool)  [unwired: 8 in, 1 out]
                  n271 = Number To Fractional String(number=w966, width (-)=i16 3 ("Breite (-)"), precision (6)=i16 0 ("Genauigkeit (6)")) -> (F-format string=w967:string)  [unwired: 1 in]
                  n272 = Select(t=w951, s=w952, f=w950) -> (s? t:f=w949:dbl)
                  n273 = case shown="\"ppm\", Standard" w954 {
                    tunnel: [i16 1 ("Genauigkeit (6)") i16 3 ("Genauigkeit (6)")] -> w977
                    tunnel: w949 -> [w987 w992]
                    tunnel: [w987 w991] -> w978
                    tunnel: ["ppm" "%"] -> w975
                    tunnel: w950 -> [_ w989]
                    frame "ppm", Default {
                      # "ppm"
                    }
                    frame "%" {
                      n274 = disable-structure shown="Aktiviert" {
                        disable-tunnel: w992 -> [_ w997]
                        disable-tunnel: [w996 w997] -> w991
                        disable-tunnel: w989 -> [w994 _]
                        frame Disabled {
                          # "%"
                          n275 = Multiply(x=w994, y=T5 10000.0) -> (x*y=w996:dbl)
                        }
                        frame Enabled {
                        }
                      }
                    }
                  }
                  n276 = Number To Decimal String(number=w965) -> (decimal integer string=w973:string)  [unwired: 1 in]
                  n277 = case shown="\"CH4\"" w958 {
                    tunnel: ["2" "3" "4" "5" "7" "1" "1"] -> w968
                    frame "CO2" {
                    }
                    frame "O2" {
                    }
                    frame "CH4" {
                    }
                    frame "C3H8" {
                    }
                    frame "NO" {
                    }
                    frame "0", Default {
                    }
                    frame "CO" {
                    }
                  }
                  n278 = Number To Fractional String(use system decimal point (T)=FALSE ("Systemdezimalzeichen verwenden (T)"), number=w978, precision (6)=w977) -> (F-format string=w974:string)  [unwired: 1 in]
                  n279 = Build Array(w968, w973, w967, w974, w975) -> (w971:string[])
                  n280 = call "GDC Kom.vi"("Befehl"=Aktion_Befehl."GD parameter", "Daten"=w971) -> ("Status (alarm)"=w960:bool, "Fehler"=w961:bool, "Status"=w964:string)  [unwired: 3 in, 4 out]
                  n281 = call "Map GD Errors.vi"("Störung Gasteiler"=w960, "Error"=T33 {"Pressure carrier gas"=FALSE, "Pressure diluted gas"=FALSE, "Outlet Pressure"=FALSE, "SNOX before SAIR"=FALSE}, "Störung Kommunikation"=w961) -> ("LIN Errors-Cluster (Ausgang)"=w963:T29)  [unwired: 7 in, 1 out]
                }
                frame #1 {
                  n282 = call "GDC Kom.vi"("Befehl"=Aktion_Befehl."Info") -> ("Gas"=w1000:string[], "Konzentration 2"=w999:string)  [unwired: 4 in, 5 out]
                  n283 = Build Array (concatenate)(w1000, w999) -> (w998:string[])
                }
                frame #2 {
                  n284 = Increment(x=w1020) -> (x+1=w1021:T25)
                  n285 = Multiply(x=0.9, y=w1021) -> (x*y=w1024:dbl)
                  n286 = call "Stufen gleichmäßig aufteilen.vi"("Punkte umkehren"=w1018, "Stufen"=w1019, "Anzahl"=w1021) -> ("Stufen"=w1022:u16[])  [unwired: 8 in]
                  n287 = Round Toward -Infinity(1:w1024) -> (0:w1025:dbl)
                  n288 = Index Array(array=w1006, index=w1005) -> (element=w1007:dbl)
                  n289 = To Long Integer(number=w1025) -> (32bit integer=w1023:i32)
                  n290 = Build Array (concatenate)(w1017, w1006) -> (w1012:dbl[])
                  n291 = for {
                    tunnel: [w1042] -> w1009 mode=indexing
                    tunnel: w1023 -> [w1047]
                    tunnel: w1022 -> [w1044] mode=indexing
                    tunnel: [w1034] -> w1013 mode=indexing
                    tunnel: w1019 -> [w1032]
                    i -> [w1033]
                    stop <- w1041 stop-if-true
                    # "#GDC-One_Zeitverzögerung_Stufenabfrage"
                    n292 = Decrement(x=w1032) -> (x-1=w1028:T5)
                    n293 = Equal?(x=0, y=w1033) -> (x = y?=w1030:bool)
                    n294 = Equal?(x=w1028, y=w1033) -> (x = y?=w1031:bool)
                    n295 = Or(x=w1031, y=w1030) -> (x .or. y?=w1029:bool)
                    n296 = case shown="False" w1029 {
                      tunnel: w1047 -> [w1050 _]
                      tunnel: [w1049 w1052] -> w1046
                      tunnel: w1044 -> [w1048 w1052]
                      frame False {
                        n297 = In Range and Coerce(upper limit=w1050, x=w1048, lower limit=0) -> (coerced(x)=w1049:i32)  [unwired: 1 out]
                      }
                      frame True {
                      }
                    }
                    n298 = Number To Decimal String(number=w1046, width (-)=i16 3 ("Breite (-)")) -> (decimal integer string=w1035:string)
                    n299 = call <vilib>:"Space Constant.vi"() -> ("String"=w1038:string)
                    n300 = Search and Replace String(replace all?=TRUE ("Alle ersetzen? (F)"), input string=w1035, search string=w1038, replace string="0" ("Ersetzungs-String (\"\")")) -> (result string=w1034:string)  [unwired: 4 in, 3 out]
                    n301 = Wait (ms)(milliseconds to wait=u32 200 ("Zu wartende ms")) -> ()  [unwired: 1 out]
                    n302 = Build Array(w1034) -> (w1043:string[])
                    n303 = call "GDC Kom.vi"("Befehl"=Aktion_Befehl."GD point", "Daten"=w1043) -> ("Status (alarm)"=w1041:bool, "Konzentration"=w1042:string)  [unwired: 3 in, 5 out]
                  }
                  n304 = call "GD_MG_MagicFormula_OnOff.vi"("Aktion"=enum16{"lesen", "schreiben", "init"}."lesen") -> ("MG_use_magic_formula"=w1008:bool)  [unwired: 8 in, 1 out]
                  n305 = Build Array (concatenate)(w1016, w1015) -> (w1011:string[])
                  n306 = Select(t=w1004, s=w1008, f=w1007) -> (s? t:f=w1003:dbl)
                  n307 = call "GD_GesamtKonz_back_calc.vi"("ohne Einheiten"=TRUE, "Gesamtkonzentration"=w1003, "Einheiten"=w1011, "Konzentration der Komponenten"=w1012, "Stufen"=w1009, "Punkte (Eingang)"=w1013) -> ("Stufentabellen (Ausgang)"=w1014:string[][][])  [unwired: 4 in, 1 out]
                }
                frame #3 {
                  n308 = call "GDC Kom.vi"("Befehl"=Aktion_Befehl."Standby") -> ()  [unwired: 4 in, 7 out]
                }
              }
            }
            frame 4 {
              # "HovaCAL #Option10xSpanAuto\nwird in HavaCAL Komm gemacht,\naber damit man es sieht ?"
              n309 = Index Array(array=w1071, index=w1059) -> (element=w1070:cluster{"Komponente:":T8, "Konzentration":dbl})
              n310 = Index Array(array=w1060, index=w1059) -> (element=w1055:dbl)
              n311 = call "GD_MG_MagicFormula_OnOff.vi"("Aktion"=enum16{"lesen", "schreiben", "init"}."lesen") -> ("MG_use_magic_formula"=w1058:bool)  [unwired: 8 in, 1 out]
              n312 = Build Array (concatenate)(w1068, w1060) -> (w1061:dbl[])
              n313 = Select(t=w1056, s=w1058, f=w1055) -> (s? t:f=w1057:dbl)
              n314 = Build Array (concatenate)(w1067, w1066) -> (w1062:string[])
              n315 = Bundle By Name(cluster=w1070, "Konzentration"=w1057) -> (w1069:cluster{"Komponente:":T8, "Konzentration":dbl})
              n316 = disable-structure shown="Aktiviert" {
                disable-tunnel: [w1079 w1085] -> w1077
                disable-tunnel: [w1078 w1084] -> w1076
                disable-tunnel: w1069 -> [_ w1083]
                disable-tunnel: w1074 -> [_ w1082]
                disable-tunnel: w1073 -> [_ w1081]
                disable-tunnel: w1072 -> [_ w1080]
                frame Disabled {
                  n317 = call "HovaCal Stufen aufteilen.vi"() -> (1:"Stufen"=w1078:dbl[], 3:"Stufen"=w1079:u16[])  [unwired: 8 in, 2 out]
                }
                frame Enabled {
                  n318 = call "HovaCal Stufen aufteilen.vi"("Komponentenauswahl"=w1083, "Punkte umkehren"=w1080, "Anzahl Stufen"=w1081, "Gasteiler Stufen"=w1082) -> (1:"Stufen"=w1084:dbl[], 3:"Stufen"=w1085:u16[])  [unwired: 4 in, 2 out]
                }
              }
              n319 = Number To Fractional String(number=w1076, precision (6)=i16 2 ("Genauigkeit (6)")) -> (F-format string=w1063:string[])  [unwired: 2 in]
              n320 = Number To Decimal String(number=w1077) -> (decimal integer string=w1064:string[])  [unwired: 1 in]
              n321 = call "GD_GesamtKonz_back_calc.vi"("Gesamtkonzentration"=w1057, "Einheiten"=w1062, "Konzentration der Komponenten"=w1061, "Stufen"=w1063, "Punkte (Eingang)"=w1064) -> ("Stufentabellen (Ausgang)"=w1065:string[][][])  [unwired: 5 in, 1 out]
            }
            frame 5 {
              # "Horiba 710 c ... manuell !"
              n322 = Index Array(array=w1090, index=w1089) -> (element=w1088:dbl)
              n323 = call "FGV Gasteilerkorrektur.vi"("Aktion"=Aktion_FGV_Gasteiler_Korrektur."Vereinzeln") -> ("Vereinzelt"=w1107:sgl[], "Aktiv"=w1105:bool)  [unwired: 9 in, 4 out]
              n324 = Divide(x=w1107, y=100.0) -> (x/y=w1104:dbl[])
              n325 = call "GD_MG_MagicFormula_OnOff.vi"("Aktion"=enum16{"lesen", "schreiben", "init"}."lesen") -> ("MG_use_magic_formula"=w1092:bool)  [unwired: 8 in, 1 out]
              n326 = Build Array (concatenate)(w1100, w1090) -> (w1094:dbl[])
              n327 = case shown="True" w1105 {
                tunnel: dbl[] [0.0, 0.1, 0.2, 0.3, 0.4, 0.5, 0.6, 0.7, 0.8, 0.9, 1.0] -> [w1115 w1119]
                tunnel: w1104 -> [_ w1117]
                tunnel: [w1115 w1118] -> w1103
                frame False {
                }
                frame True {
                  n328 = Reverse 1D Array(array=w1117) -> (reversed array=w1116:dbl[])
                  n329 = Add(x=w1119, y=w1116) -> (x+y=w1118:dbl[])
                }
              }
              n330 = Select(t=w1091, s=w1092, f=w1088) -> (s? t:f=w1087:dbl)
              n331 = Build Array (concatenate)(w1098, w1099) -> (w1093:string[])
              n332 = Multiply(x=w1103, y=w1087) -> (x*y=w1112:dbl[])
              n333 = call "Stellengenauigkeit.vi"("Genauigkeit (6)"=i16 5) -> ("Formatstring"=w1113:string)  [unwired: 9 in, 1 out]
              n334 = for {
                tunnel: w1113 -> [w1126]
                tunnel: w1112 -> [w1125] mode=indexing
                tunnel: [w1120] -> w1109 mode=indexing
                tunnel: [w1124] -> w1111 mode=indexing
                i -> [w1124]
                n335 = Format Value(format string=w1126, value (0)=w1125) -> (output string=w1121:string)  [unwired: 1 in]
                n336 = Search and Replace String(input string=w1121, search string="," ("Such-String"), replace string="." ("Ersetzungs-String (\"\")")) -> (result string=w1120:string)  [unwired: 5 in, 3 out]
              }
              n337 = Number To Decimal String(number=w1111) -> (decimal integer string=w1110:string[])  [unwired: 1 in]
              n338 = case shown="True" w1101 {
                tunnel: w1110 -> [w1128 w1132]
                tunnel: [w1128 w1131] -> w1097
                tunnel: w1109 -> [w1127 w1130]
                tunnel: [w1127 w1129] -> w1095
                frame False {
                }
                frame True {
                  n339 = Reverse 1D Array(array=w1132) -> (reversed array=w1131:string[])
                  n340 = Reverse 1D Array(array=w1130) -> (reversed array=w1129:string[])
                }
              }
              n341 = call "GD_GesamtKonz_back_calc.vi"("Gesamtkonzentration"=w1087, "Einheiten"=w1093, "Konzentration der Komponenten"=w1094, "Stufen"=w1095, "Punkte (Eingang)"=w1097) -> ("Stufentabellen (Ausgang)"=w1096:string[][][])  [unwired: 5 in, 1 out]
            }
          }
          n342 = call "GD TimeStamp.vi"() -> ("date/time string"=w523:string)  [unwired: 10 in, 1 out]
          n343 = Bundle By Name(cluster=T28 {"Wobei"="", "Status"="", "Errors"={"Störung Kommunikation"=FALSE, "Pressure carrier gas"=FALSE, "Pressure diluted gas"=FALSE, "Outlet Pressure"=FALSE, "SNOX before SAIR"=FALSE, "Störung Gasteiler"=FALSE}, "Empfangsdaten"=[], "Zeitstempel"=""} ("GD Info-Cluster"), "Zeitstempel"=w523, "Wobei"="GD get Table of Points" ("Status"), "Status"=w542, "Errors"=w541, "Empfangsdaten"=w540) -> (w539:T28)
          n344 = case shown="True" w538 {
            tunnel: w539 -> [_ w1136]
            tunnel: w537 -> [_ w1133]
            frame False {
            }
            frame True {
              n345 = call "Status mit GD Info aktualisieren.vi"("show Status even if no Error"=TRUE, "Sprachliste"=w1133, "GD Info-Cluster in"=w1136) -> ("Status out"=→"Status out":string)  [unwired: 7 in, 1 out]
            }
          }
          n346 = call "FGV GD Errors sammeln.vi"("Aktion"=Aktion_FGV_GD_Errors_sammeln."GD Infos sammeln", "GD Info-Cluster in"=w539) -> ()  [unwired: 7 in, 3 out]
        }
        frame True {
          # "Wenn 0 (----) kommt dann nicht abfragen"
        }
      }
    }
  }
  n347 = Decrement(x=w8) -> (x-1=→"Komponente out":T8)
  n348 = Bundle By Name(cluster=T4 {"Stufen Tabellen out"=[], "EGAK"=[], "AGAK"=[]} ("GD out"), "Stufen Tabellen out"=w43, "EGAK"=w42, "AGAK"=w44) -> (→"GD out":T4)
  "error out" <- "error in (no error)"
